vi "GTcode_v6.vi"() -> ()   [LabVIEW 2016]
uses:
  <vilib>/Utility/error.llb/DialogType.ctl
  <vilib>/Analysis/5stat.llb/RMS (DBL).vi
  <vilib>/Utility/config.llb/Write Key (String).vi
  <vilib>/Utility/config.llb/Write Key (U32).vi
  <vilib>/Utility/config.llb/Write Key (Double).vi
  <vilib>/Utility/config.llb/Write Key (I32).vi
  <vilib>/Utility/config.llb/Read Key (U32).vi
  <vilib>/Utility/config.llb/Read Key (I32).vi
  <vilib>/Waveform/WDTFileIO.llb/ Write Waveform to File.vi
  <vilib>/Waveform/WDTOps.llb/WDT Append Waveforms DBL.vi
  DCScode_simulISS_MAP/flex05-4chPascal.dll
  <vilib>/Utility/config.llb/NI_LVConfig.lvlib
  DCScode_simulISS_MAP/flex05oem8chauto100nsPASCAL_win7.dll
  <vilib>/Analysis/NI_AALBase.lvlib
  <vilib>/Analysis/NI_AALPro.lvlib
  <resource>/objmgr/daqmx.rc
panel:
  in  "Tab Control":T1(tab)=enum."Real Time Fitting Parameters"
  out "mean":dbl format="%0.1e"
  out "COV":dbl format="%0.1f"
  in  "Fixed Time":bool
  in  "Detector Used":T2(ring)=enum."Det 2"
  in  "Real Time Fitting?":bool=TRUE
  out "g2":cluster{"Delay Time":sgl[], sgl[]}[](graph) caption="Normalized Correlation Function"
  out "Tau":cluster{"tmp":dbl, dbl}(graph) caption="Relative Changes of Flow"
  in  "QUIT":bool
  in  "Clear plots":bool
  in  "Baseline":bool
  in  "MARK\nMark":bool
  in  "Stop":bool
  in  "Sequence Scan":bool
  out "Mark #":u32
  out "Trial #":u32
  out "Frame #":u32
  out "Det 8":sgl format="%.3f"
  out "Det 7":sgl format="%.3f"
  out "Det 6":sgl format="%.3f"
  out "Det 5":sgl format="%.3f"
  out "Det 4":sgl format="%.3f"
  out "Det 3":sgl format="%.3f"
  out "Det 2":sgl format="%.3f"
  out "Det 1":sgl format="%.3f"
  out "Computer Time":string="2010-1-12 23:16:10"
  in  "D1":bool
  in  "D2":bool
  in  "D3":bool
  in  "D4":bool
  in  "D5":bool
  in  "D6":bool
  in  "D7":bool
  in  "D8":bool
  out "Tau 2":T3(graph)={1.6593152555505744e-08, 3.9427894777554196e-08, 4.065716407938411e-08, 1.5135790977358522e-08, 2.4870420100428357e-08, 7.094765128107397e-08, 0.0, 4.1348620928852906e-07, 1.5886917674344795e-08, 4.0280526032721455e-08, -1.0, -1.0} caption="Blood Flow Index (cm2/s)"
  in  "Fixed # of Frames":u32=5
  out "Status":string="Quit"
  in  "Optical Switch OPEN":bool
  in  "Delay between frames(ms)":u32=500
  out "Time Left (ms)":sgl format="%.3f"
  in  "Integration Time (ms)":sgl=1000.0 min=1 max=13000 step=1
  in  "File\nName:":string="test0"
  in  "Data Save Directory:":path=path "C:/data"
  in  "ISS Lasers ON":bool
  in  "Test":bool=TRUE
  out "Moving Avg RMS":dbl(slide) scale=0.0..0.07
  out "Moving Avg RMS Graph":dbl(graph)
  out "raw data":dynamicdata(graph)
  out "Trial Data 2":waveform(dbl)(graph)
  out "Reset Data Acquisition\nAnd UI Updating":bool=TRUE
  out "Trial In Progress":bool
  in  "Lines":tag="Dev1/port1/line0:1, Dev1/port1/line3:7"
  in  "Delaytime(ms)":u32=200
  in  "Initialize Correlator":bool
  in  "Detector Select":enum32{"4 Detectors", "8 Detectors"}(radio)=enum."8 Detectors"
  in  "Update Time (ms)\nDO NOT CHANGE!":u32=105 min=1 max=999 step=1
  in  "Laser Input Name":refnum<visa-resource-name>="COM7"
  out "Flow in each detector":dbl[](array[numeric])=[-1.0, -1.0, -1.0, -1.0, -1.0, -1.0, -1.0, -1.0, -1.0, -1.0, -1.0, -1.0]
  in  "Visible Averages":bool[](array[boolean])=[FALSE, FALSE, FALSE, FALSE]
  in  "Avg":bool[][](array[boolean])=[[FALSE, FALSE, FALSE, FALSE, FALSE, FALSE, FALSE, FALSE], [FALSE, FALSE, FALSE, FALSE, FALSE, FALSE, FALSE, FALSE], [FALSE, FALSE, FALSE, FALSE, FALSE, FALSE, FALSE, FALSE], [FALSE, FALSE, FALSE, FALSE, FALSE, FALSE, FALSE, FALSE]]
  in  "rho":dbl[](array[numeric])=[2.5, 2.5, 2.5, 2.5, 2.5, 2.5, 2.5, 2.5, -1.0, -1.0, -1.0, -1.0]
  in  "Other Settings":u32[](array[numeric])=[1, 120, 0, 1] caption="Flow in each detector"
  in  "Initial Guess":dbl[](array[numeric])=[1e-08, 0.5, 0.05, 10.0] caption="Flow in each detector"
  out "Filtered data":waveform(dbl)
  out "Aggregate Data":waveform(dbl)[](array[waveform])
  in  "VR Data Input File":path
  in  "Trial Number":dbl
  in  "Target Percentage":dbl
  in  "VR Percent Path":path
  out "Trial Data":waveform(dbl)
  out "Rectified Moving Average Sample":waveform(dbl)[](graph)
  out "Bufffer Index":dbl
  out "Frames in Buffer":dbl
  out "Samples per frame":dbl
  in  "Lower Cut-Off":dbl=20.0
  in  "Upper Cut-Off (Not In Use)":dbl=300.0 caption="Upper Cut-Off"
  in  "File Name:":string="test0"
  in  "Sample rate (Hz)":dbl=2000.0
  in  "Frames Per Second":dbl=30.0
  in  "Moving Average Length (s)":dbl=0.5
  in  "EMG Input Device\nProduct Type":string
  out "4CH?":bool
  out "Detector#":u32=1
  out "Source#":u32=1
  # "Jake Test Version"
  # "kHz"
  # "kHz"
  # "Don't Change these Parameters unless you know clearly what you are doing"
  # "ISS Triggers Setup"
  # "Channel Parameters"
  # "Step1"
  # "Line"
  # "0"
  # "1"
  # "3"
  # "4"
  # "5"
  # "6"
  # "7"
  # "*The number of lines in the list must\nmatch the number of elements in\nthe array."
  # "Step2"
  # "Line"
  # "0"
  # "1"
  # "3"
  # "4"
  # "5"
  # "6"
  # "7"
  # "Step3"
  # "Line"
  # "0"
  # "1"
  # "3"
  # "4"
  # "5"
  # "6"
  # "7"
  # "Line    Signal\n\n0           ISS Trigger (0: OFF, 1: ON)\n1           Flow Laser 1 ON/OFF (0:OFF, 1:ON)\n2           ISS Data Acquisition (0: DONE, 1: NO)\n3           ISS Laser ON/OFF (0: ON, 1: OFF)\n4           Trigger for Marks  (0: OFF, 1: ON)\n5           Flow Laser 2 ON/OFF (0:OFF, 1:ON)\n6           Reserved\n7           Reserved"
  # "Wait ISS Data Acuisition DONE Signal"
  # "Step4"
  # "Step5"
  # "Line"
  # "0"
  # "1"
  # "3"
  # "4"
  # "5"
  # "6"
  # "7"
  # "Flow Lasers Setup"
  # "FROM FRONT PANEL"
  # "Line"
  # "0"
  # "1"
  # "3"
  # "4"
  # "5"
  # "6"
  # "7"
  # "Line"
  # "0"
  # "1"
  # "3"
  # "4"
  # "5"
  # "6"
  # "7"
  # "Det 1"
  # "Det 2"
  # "Det 3"
  # "Det 4"
  # "Det 5"
  # "Det 6"
  # "Det 7"
  # "Det 8"
  # "Avg 1"
  # "Avg 2"
  # "Avg 3"
  # "Avg 4"
  # "Db"
  # "Beta"
  # "Mua"
  # "MuS'"
  # "1"
  # "2"
  # "3"
  # "4"
  # "5"
  # "6"
  # "7"
  # "8"
  # "Avg 1"
  # "Starting Pt"
  # "End Pt"
  # "Approximate"
  # "Variables"
  # "Avg 2"
  # "Avg 3"
  # "Avg 4"
  # "Source Detector  Separations"
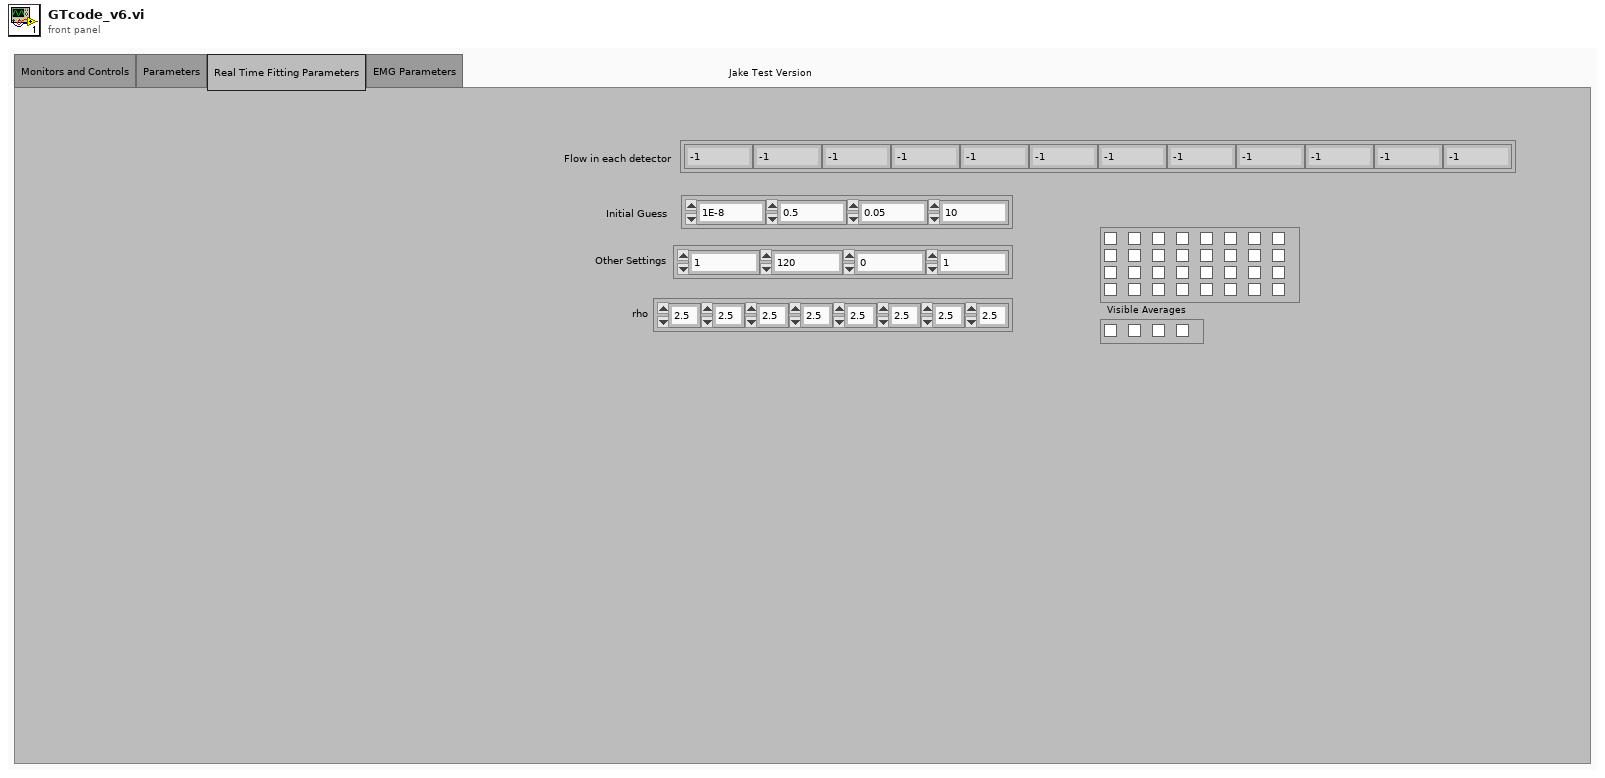
[diagram p1: front panel]
types:
  T1 = enum32{"Monitors and Controls", "Parameters", "Real Time Fitting Parameters", "EMG Parameters"}
  T2 = enum16{"Det 1", "Det 2", "Det 3", "Det 4", "Det 5", "Det 6", "Det 7", "Det 8"}
  T3 = cluster{dbl, dbl, dbl, dbl, dbl, dbl, dbl, dbl, dbl, dbl, dbl, dbl}
  T4 = typedef "DialogType.ctl" = u16
  T5 = enum8{"Enabled", "Disabled", "Disabled and Grayed Out"}
  T6 = cluster{dbl, dbl, dbl, dbl, dbl, dbl, dbl, dbl, dbl, dbl, dbl, dbl}[]
  T7 = typedef "NI_LVConfig.lvlib/Config Data RefNum.ctl" = refnum<k1>
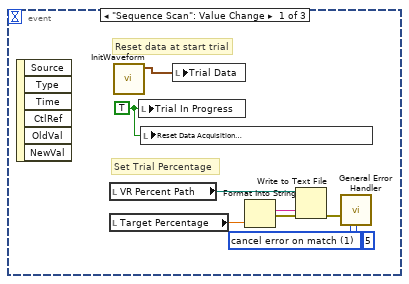
[diagram p2: hidden frame]
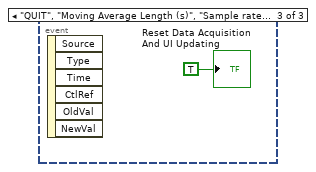
[diagram p5: hidden frame]
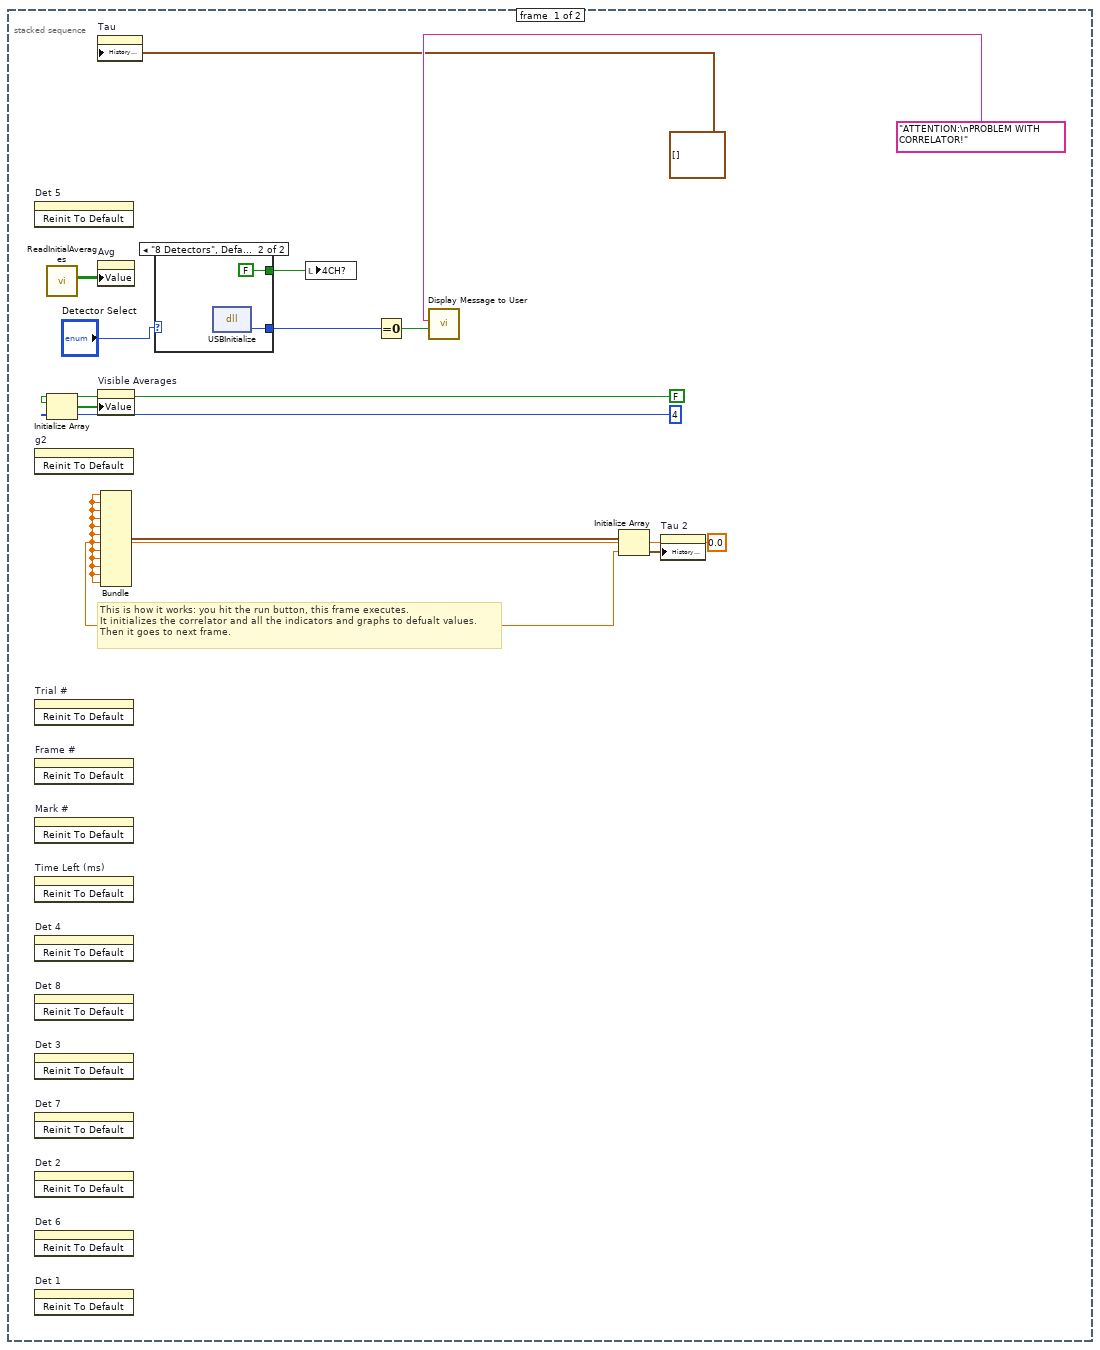
[diagram p7: hidden frame]
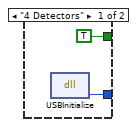
[diagram p8: hidden frame]
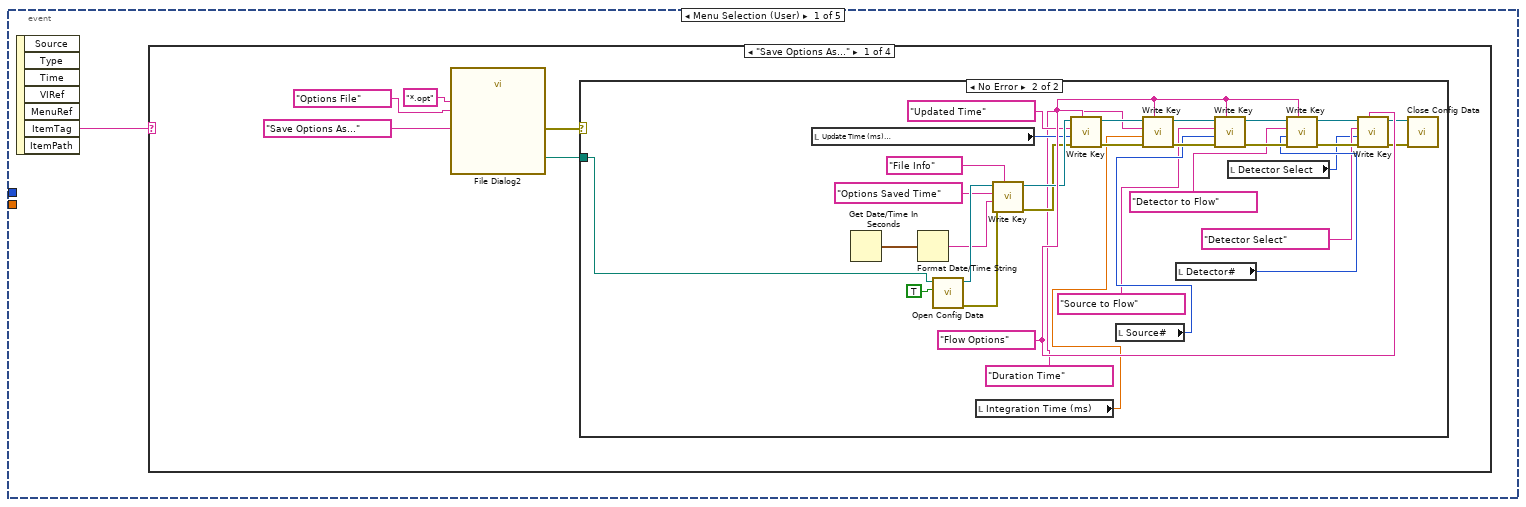
[diagram p10: hidden frame]
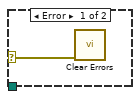
[diagram p11: hidden frame]
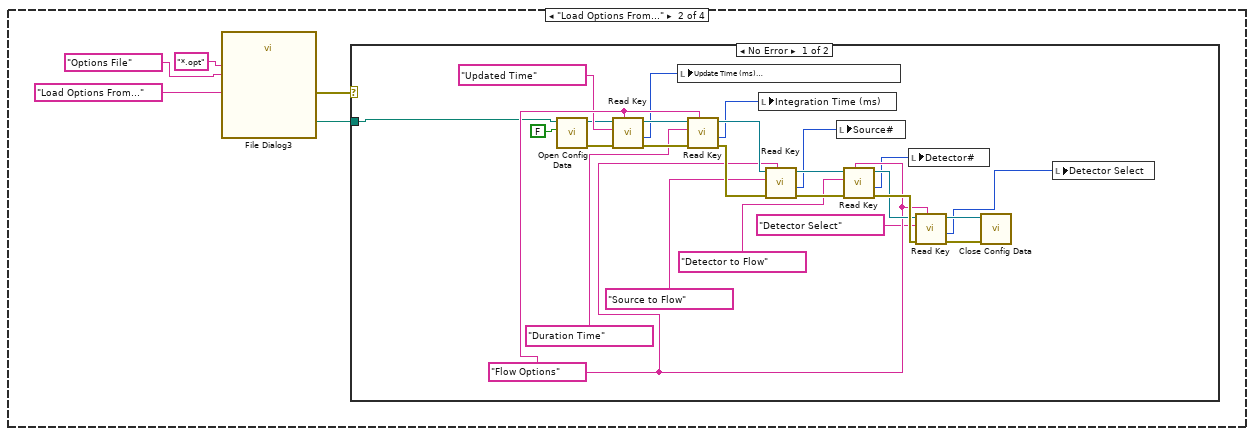
[diagram p12: hidden frame]
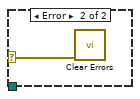
[diagram p13: hidden frame]
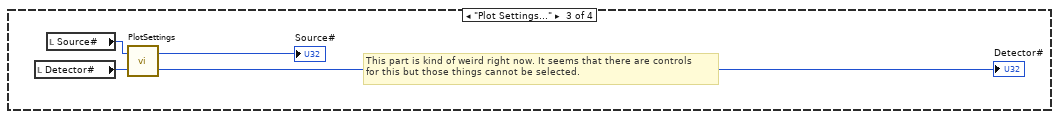
[diagram p14: hidden frame]
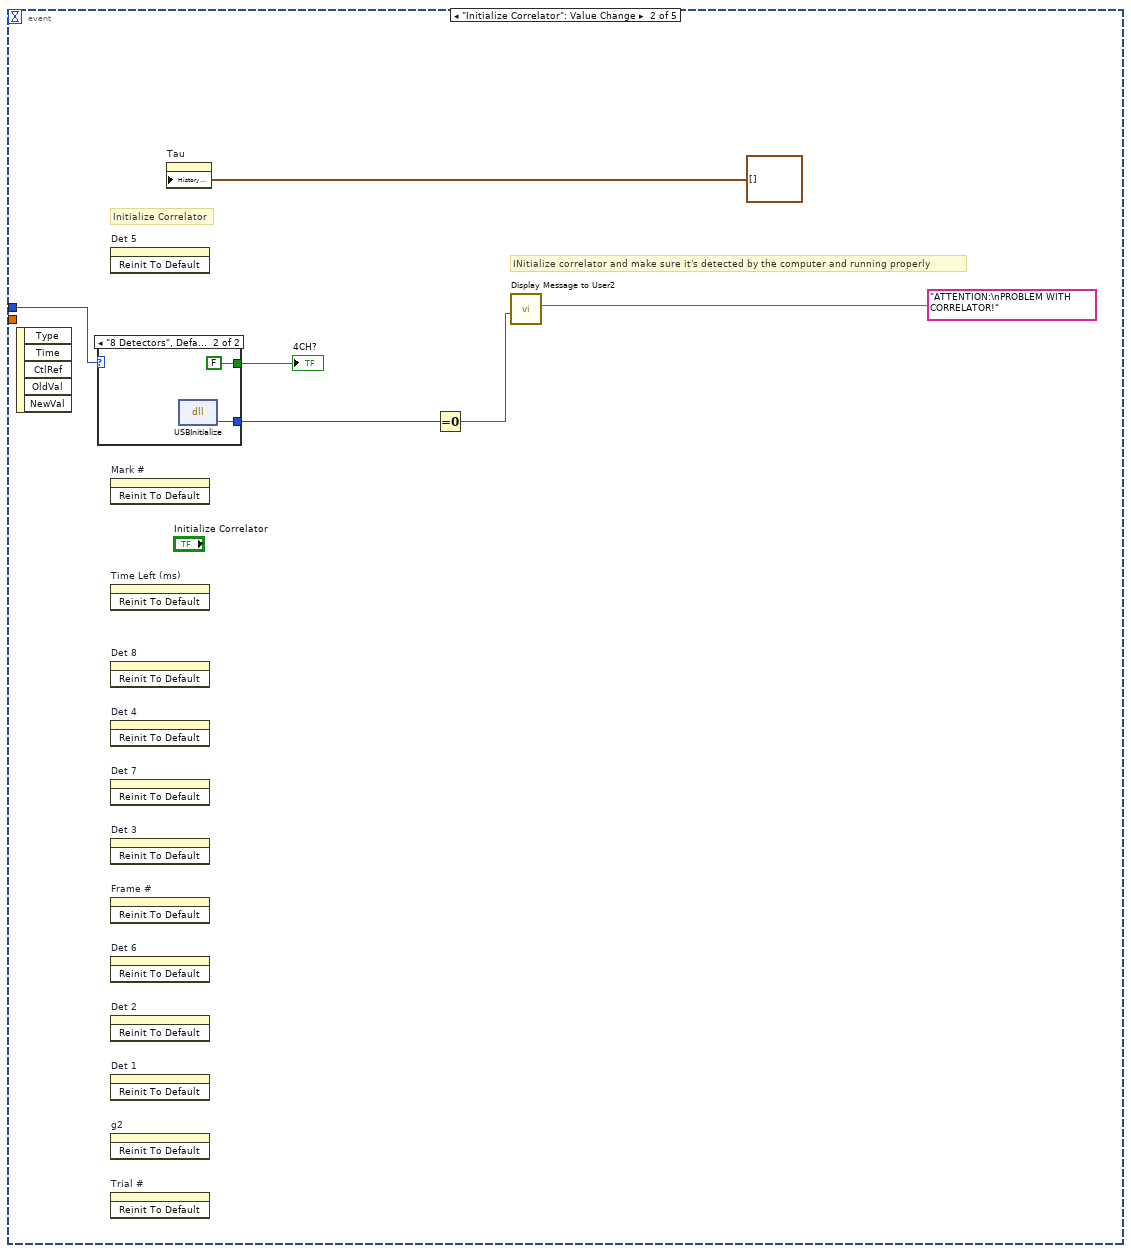
[diagram p16: hidden frame]
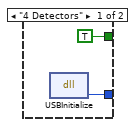
[diagram p17: hidden frame]
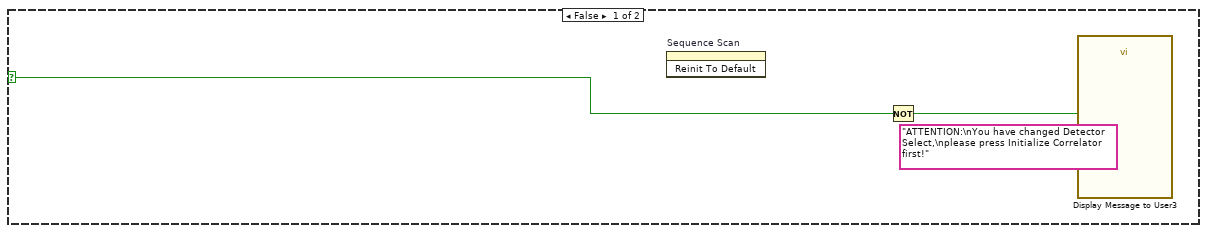
[diagram p18: hidden frame]
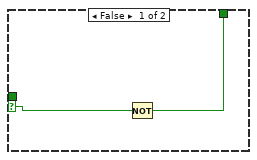
[diagram p19: hidden frame]
diagram:
  # "Where VR knows\n to look for data"
  n1 = property class="DAQmx System"() -> ("DevNames"=w2:tag[])  [unwired: 2 in, 2 out]
  n2 = for {
    tunnel: w2 -> [w6] mode=indexing
    tunnel: [w6] -> w1
    stop <- w7 stop-if-true
    n3 = property class="DAQmx Device" props=["Active Device", "ProductType", "ProductNum"]("Active Device"=w6) -> ("ProductType"=w9:string)  [unwired: 2 in, 3 out]
    n4 = Equal?(x=w9, y="EMG Input Device\nProduct Type") -> (x = y?=w7:bool)
  }
  n5 = while {
    tunnel: w1 -> [w10]
    stop <- w11 stop-if-true
    # "Initialize Stuff"
    # "Listen for settings changes and restart runtime loop\nAlso make updates for trial changes"
    n6 = while {
      tunnel: w10 -> [w62]
      stop <- w65 stop-if-true
      n7 = local read "Sample rate (Hz)"() -> (w79:dbl)
      n8 = local read "Samples per frame"() -> (w78:dbl)
      n9 = local read "Reset Data Acquisition\nAnd UI Updating"() -> (w64:bool)
      n10 = local read "raw data"() -> (w76:dynamicdata)
      n11 = local read "Aggregate Data"() -> (w72:waveform(dbl)[])
      n12 = local read "Filtered data"() -> (w71:waveform(dbl))
      n13 = local read "Bufffer Index"() -> (w70:dbl)
      n14 = local read "Frames in Buffer"() -> (w67:dbl)
      n15 = local read "Trial In Progress"() -> (w63:bool)
      n16 = local read "Reset Data Acquisition\nAnd UI Updating"() -> (w65:bool)
      n17 = case shown="True" w63 {
        frame False {
        }
        frame True {
          # "Start aggregating data for trial"
          n18 = local read "Filtered data"() -> (w81:waveform(dbl))
          n19 = local read "Trial Data"() -> (w82:waveform(dbl))
          n20 = call-poly <vilib>:"Append Waveforms.vi"("waveform B"=w81, "waveform A"=w82) -> ("waveform out"=w80:waveform(dbl))  [unwired: 8 in, 1 out]
          n21 = local write "Trial Data"(w80) -> ()
        }
      }
      n22 = call "Filter"("Lower Cut-Off"="Lower Cut-Off", "Signal"=w76) -> ("Filtered Signal"=w74:dynamicdata)  [unwired: 8 in, 1 out]
      n23 = Increment(x=w70) -> (x+1=w66:dbl)
      n24 = Replace Array Subset(array=w72, new element=w71, index=w70) -> (w69:waveform(dbl)[])
      n25 = call "DAQ Assistant8"("rate"=w79, "number of samples"=w78, "stop (T)"=w64, "device name"=w62) -> ("data"=→"raw data":dynamicdata)  [unwired: 13 in, 2 out]
      n26 = Quotient & Remainder(x=w66, y=w67) -> (x-y*floor(x/y)=w68:dbl)  [unwired: 1 out]
      n27 = local write "Aggregate Data"(w69) -> ()
      n28 = call "Convert from Dynamic Data"("Dynamic Data Type"=w74) -> ("Waveform"=→"Filtered data":waveform(dbl))  [unwired: 3 in]
      n29 = local write "Bufffer Index"(w68) -> ()
    }
    n30 = local read "Moving Average Length (s)"() -> (w17:dbl)
    n31 = local read "Frames Per Second"() -> (w16:dbl)
    n32 = local read "QUIT"() -> (w11:bool)
    n33 = local read "Sample rate (Hz)"() -> (w20:dbl)
    n34 = local read "Frames Per Second"() -> (w19:dbl)
    n35 = local write "Reset Data Acquisition\nAnd UI Updating"(FALSE) -> ()
    n36 = Divide(x=w20, y=w19) -> (x/y=→"Samples per frame":dbl)
    n37 = Multiply(x=w17, y=w16) -> (x*y=w12:dbl)
    "Frames in Buffer" <- w12
    n38 = call "CreateWaveformArray.vi"("bufferSize"=w12) -> ("initialized array"=→"Aggregate Data":waveform(dbl)[])  [unwired: 5 in, 1 out]
    n39 = event shown="[1] \"Stop\": Value Change" {
      selector: _ -> [_ _ _]
      dyn-events: _ -> [_ _ _]
      timeout: _ -> [_ _ _]
      event "Sequence Scan": Value Change {
        w27 = 1 items=["no exception", "cancel error on match", "set error on match"] ("[exception action] (none:0)")
        w28 = TRUE ("Trial In Progress")
        # "Set Trial Percentage"
        # "Reset data at start trial"
        n40 = event-data() -> ()  [unwired: 1 in, 6 out]
        n41 = local read "VR Percent Path"() -> (w22:path)
        n42 = local read "Target Percentage"() -> (w21:dbl)
        n43 = call "InitWaveform.vi"() -> ("output waveform"=w29:waveform(dbl))  [unwired: 11 in]
        n44 = local write "Trial In Progress"(w28) -> ()
        n45 = local write "Reset Data Acquisition\nAnd UI Updating"(w28) -> ()
        n46 = local write "Trial Data"(w29) -> ()
        n47 = Format Into String(w21) -> (resulting string=w23:string, error out=w24:errorcluster)  [unwired: 3 in]
        n48 = Write to Text File(file (use dialog)=w22, text=w23, error in=w24) -> (error out=w25:errorcluster)  [unwired: 1 in, 2 out]
        n49 = call <vilib>:"General Error Handler.vi"("error in (no error)"=w25, "[exception action] (none:0)"=w27, "[exception code]"=5) -> ()  [unwired: 8 in, 5 out]
      }
      event "Stop": Value Change {
        # "Only Execute if Trial Already in progress"
        n50 = event-data() -> ()  [unwired: 1 in, 6 out]
        n51 = local read "Trial In Progress"() -> (w30:bool)
        n52 = case shown="True" w30 {
          frame False {
          }
          frame True {
            w31 = T4 2 items=["no dialog", "OK message", "continue or stop message", "OK message + warnings", "continue/stop + warnings"] ("type of dialog (OK msg:1)")
            w33 = 1 items=["no exception", "cancel error on match", "set error on match"] ("[exception action] (none:0)")
            # "End Trial and save data, create directory if needed"
            n53 = local read "Data Save Directory:"() -> (w38:path)
            n54 = local read "Trial Data"() -> (w45:waveform(dbl))
            n55 = local read "File Name:"() -> (w37:string)
            n56 = local write "Trial In Progress"(FALSE ("Trial In Progress")) -> ()
            n57 = local write "Reset Data Acquisition\nAnd UI Updating"(TRUE ("Reset Data Acquisition\nAnd UI Updating")) -> ()
            n58 = Concatenate Strings(w37, "_EMG.dat" ("string")) -> (w35:string)
            n59 = call <vilib>:"Check if File or Folder Exists.vi"("path"=w38) -> ("file or folder exists?"=w42:bool, "dup path"=w40:path)  [unwired: 8 in, 1 out]
            n60 = case shown="False" w42 {
              tunnel: [w47 w49] -> w41
              tunnel: w40 -> [w48 w49]
              frame False {
                n61 = Create Folder(path (use dialog)=w48) -> (created path=w47:path)  [unwired: 2 in, 2 out]
              }
              frame True {
              }
            }
            n62 = Build Path(base path=w41, name or relative path=w35) -> (appended path=w39:path)
            n63 = call-poly <vilib>:"Write Waveforms to File.vi"("append to file? (new file:F)"=FALSE, "waveform"=w45, "file path (dialog if empty)"=w39) -> ("error out"=w32:errorcluster)  [unwired: 7 in, 1 out]
            n64 = call <vilib>:"General Error Handler.vi"("type of dialog (OK msg:1)"=w31, "error in (no error)"=w32, "[exception action] (none:0)"=w33, "[exception code]"=1430) -> ()  [unwired: 7 in, 5 out]
          }
        }
      }
      event "QUIT", "Moving Average Length (s)", "Sample rate (Hz)", "Frames Per Second": Value Change {
        n65 = event-data() -> ()  [unwired: 1 in, 6 out]
        "Reset Data Acquisition\nAnd UI Updating" <- TRUE
      }
    }
    n66 = while {
      stop <- w61 stop-if-true
      # "Grab Relevant Sample from Moving Average, Update UI, Save Data if necessary"
      # "Wait proper duration"
      # "Save RMS Value\nFor this Frame To VR"
      # "Display RMS Data\nTo Thermometer\nAnd Moving Avg RMS\nGraph"
      # "Grab Current Moving\nAverage and Rectify"
      # "Get Moving Average Sample"
      # "Rectify"
      n67 = local read "Rectified Moving Average Sample"() -> (w58:waveform(dbl)[])
      n68 = local read "Bufffer Index"() -> (w53:dbl)
      n69 = local read "Frames in Buffer"() -> (w52:dbl)
      n70 = local read "Aggregate Data"() -> (w51:waveform(dbl)[])
      n71 = local read "Frames Per Second"() -> (w57:dbl)
      n72 = local read "Reset Data Acquisition\nAnd UI Updating"() -> (w61:bool)
      n73 = call "FramesPerSecondTOMilliseconds.vi"("Thermometer\nFps"=w57) -> ("x*y"=w56:dbl)  [unwired: 10 in]
      n74 = call "GetSubarrayOfCircularBuffer.vi"("initialized array"=w51, "buffer size"=w52, "subset size"=w52, "start index"=w53) -> ("initialized array 2"=w54:waveform(dbl)[])  [unwired: 7 in]
      n75 = Wait (ms)(milliseconds to wait=w56) -> ()  [unwired: 1 out]
      n76 = local read "Trial Data"() -> (→"Trial Data 2":waveform(dbl))
      n77 = Absolute Value(x=w54) -> (abs(x)=→"Rectified Moving Average Sample":waveform(dbl)[])
      n78 = call-poly <vilib>:"RMS.vi"("X"=w58) -> ("rms value"=→"Moving Avg RMS" →"Moving Avg RMS Graph":dbl)  [unwired: 1 out]
    }
    "Bufffer Index" <- 0.0 ("Bufffer Index")
  }
  n79 = local read "Laser Input Name"() -> (w4:refnum<visa-resource-name>)
  n80 = call "iBs.vi"("Laser On/Off"=FALSE, "VISA resource name"=w4) -> ()
  n81 = stacked-sequence {
    frame #0 {
      w85 = 0.0
      # "This is how it works: you hit the run button, this frame executes.\nIt initializes the correlator and all the indicators and graphs to defualt values.\nThen it goes to next frame."
      n82 = invoke on="Det 5" class="DigNum (strict)" method="Reinit To Default"() -> ()  [unwired: 3 in, 3 out]
      n83 = invoke on="g2" class="XYGraph (strict)" method="Reinit To Default"() -> ()  [unwired: 3 in, 3 out]
      n84 = invoke on="Trial #" class="DigNum (strict)" method="Reinit To Default"() -> ()  [unwired: 3 in, 3 out]
      n85 = invoke on="Frame #" class="DigNum (strict)" method="Reinit To Default"() -> ()  [unwired: 3 in, 3 out]
      n86 = invoke on="Mark #" class="DigNum (strict)" method="Reinit To Default"() -> ()  [unwired: 3 in, 3 out]
      n87 = invoke on="Time Left (ms)" class="DigNum (strict)" method="Reinit To Default"() -> ()  [unwired: 3 in, 3 out]
      n88 = invoke on="Det 4" class="DigNum (strict)" method="Reinit To Default"() -> ()  [unwired: 3 in, 3 out]
      n89 = invoke on="Det 8" class="DigNum (strict)" method="Reinit To Default"() -> ()  [unwired: 3 in, 3 out]
      n90 = invoke on="Det 3" class="DigNum (strict)" method="Reinit To Default"() -> ()  [unwired: 3 in, 3 out]
      n91 = invoke on="Det 7" class="DigNum (strict)" method="Reinit To Default"() -> ()  [unwired: 3 in, 3 out]
      n92 = invoke on="Det 2" class="DigNum (strict)" method="Reinit To Default"() -> ()  [unwired: 3 in, 3 out]
      n93 = invoke on="Det 6" class="DigNum (strict)" method="Reinit To Default"() -> ()  [unwired: 3 in, 3 out]
      n94 = invoke on="Det 1" class="DigNum (strict)" method="Reinit To Default"() -> ()  [unwired: 3 in, 3 out]
      n95 = call "ReadInitialAverages.vi"() -> ("avgOut"=w84:bool[][])  [unwired: 11 in]
      n96 = Initialize Array(FALSE, 4) -> (w83:bool[])
      n97 = property on="Tau" class="WFChart (strict)"("History Data"=cluster{"tmp":dbl, dbl}[] []) -> ()  [unwired: 2 in, 2 out]
      n98 = property on="Avg" class="Arr (strict)"("Value"=w84) -> ()  [unwired: 2 in, 2 out]
      n99 = property on="Visible Averages" class="Arr (strict)"("Value"=w83) -> ()  [unwired: 2 in, 2 out]
      n100 = Bundle(w85, w85, w85, w85, w85, w85, w85, w85, w85, w85, w85, w85) -> (w87:T3)  [unwired: 1 in]
      n101 = case shown="\"8 Detectors\", Default" "Detector Select" {
        tunnel: [w97 w99] -> w95
        tunnel: [TRUE FALSE] -> w93
        frame "4 Detectors" {
          n102 = dll-call lib="C:/Users/BUCKLEY-ADMIN/Desktop/DCScode_simulISS_MAP/flex05-4chPascal.dll" fn="USBInitialize" label="InitCH4"() -> ("return type"=w97:u8)  [unwired: 3 in, 2 out]
        }
        frame "8 Detectors", Default {
          n103 = dll-call lib="C:/Users/BUCKLEY-ADMIN/Desktop/DCScode_simulISS_MAP/flex05oem8chauto100nsPASCAL_win7.dll" fn="USBInitialize" label="InitCH8"() -> ("return type"=w99:u8)  [unwired: 3 in, 2 out]
        }
      }
      n104 = local write "4CH?"(w93) -> ()
      n105 = Equal To 0?(x=w95) -> (x = 0?=w94:bool)
      n106 = call "Display Message to User"("Enable"=w94, "Message"="ATTENTION:\nPROBLEM WITH CORRELATOR!") -> ()  [unwired: 8 in, 2 out]
      n107 = Initialize Array(w87, w85) -> (w86:T6)
      n108 = property on="Tau 2" class="WFChart (strict)"("History Data"=w86) -> ()  [unwired: 2 in, 2 out]
    }
    frame #1 {
      n109 = while {
        stop <- w103 stop-if-true
        # "Looks at whether using 4 or 8 ch correlator\nGenerates time points for g2 function based on correlator"
        n110 = local read "Detector Select"() -> (w101:enum32{"4 Detectors", "8 Detectors"})
        n111 = case shown="\"8 Detectors\"" w101 {
          tunnel: [_ w104] -> w100
          frame "4 Detectors", Default {
          }
          frame "8 Detectors" {
            n112 = formula code="int i,j;\nfloat DelayTime[256];\nfloat first_delay;\n\nfirst_delay = 2E-7;\n\nfor(i=0;i<16;i++)\nDelayTime[i] = (i+1)*first_delay;\nfor(j=1;j<31;j++)\n    for(i=0;i<8;i++)\n         DelayTime[i+(j-1)*8+16] = DelayTime[(j-1)*8+16+i-1]+first_delay*pow(2,j);"() -> ("DelayTime"=w104:dbl[])
          }
        }
        n113 = event shown="[2] \"Sequence Scan\": Value Change" {
          selector: _ -> [_ _ _ _ _]
          dyn-events: _ -> [_ _ _ _ _]
          timeout: 500 -> [_ _ _ _ _]
          tunnel: w100 -> [_ _ w194 _ _]
          tunnel: [_ _ _ "QUIT" _] -> w103
          tunnel: w101 -> [_ w181 w190 w678 _]
          event Menu Selection (User) {
            n114 = event-data() -> ("ItemTag"=w105:string)  [unwired: 1 in, 6 out]
            n115 = case shown="\"Save Options As...\"" w105 {
              frame "Save Options As..." {
                n116 = call "File Dialog2"("prompt"="Save Options As...", "pattern (all files)"="*.opt", "pattern label"="Options File") -> ("selected path"=w107:path, "error out"=w106:errorcluster)  [unwired: 9 in, 2 out]
                n117 = case shown="No Error" w106 {
                  selector: w106 -> [w111 _]
                  tunnel: w107 -> [_ w142]
                  frame Error {
                    n118 = call <vilib>:"Clear Errors.vi"("error in (no error)"=w111) -> ()  [unwired: 5 in, 2 out]
                  }
                  frame No Error {
                    w129 = "Flow Options"
                    n119 = local read "Update Time (ms)\nDO NOT CHANGE!"() -> (w122:u32)
                    n120 = Get Date/Time In Seconds() -> (seconds since 1Jan1904=w128:timestamp)
                    n121 = Format Date/Time String(seconds (now)=w128) -> (date/time string=w124:string)  [unwired: 2 in]
                    n122 = call <vilib>:"Open Config Data.vi"("create file if necessary (T)"=TRUE, "configuration file path"=w142) -> ("error out"=w140:errorcluster, "refnum"=w139:T7)  [unwired: 7 in, 1 out]
                    n123 = local read "Integration Time (ms)"() -> (w120:sgl)
                    n124 = call-poly <vilib>:"Write Key.vi"("section"="File Info", "error in (no error)"=w140, "value"=w124, "key"="Options Saved Time", "refnum"=w139) -> ("error out"=w126:errorcluster, "refnum out"=w127:T7)  [unwired: 4 in, 1 out]
                    n125 = call-poly <vilib>:"Write Key.vi"("section"=w129, "error in (no error)"=w126, "value"=w122, "key"="Updated Time", "refnum"=w127) -> ("error out"=w138:errorcluster, "refnum out"=w137:T7)  [unwired: 4 in, 1 out]
                    n126 = local read "Source#"() -> (w119:u32)
                    n127 = call-poly <vilib>:"Write Key.vi"("section"=w129, "error in (no error)"=w138, "value"=w120, "key"="Duration Time", "refnum"=w137) -> ("error out"=w133:errorcluster, "refnum out"=w134:T7)  [unwired: 4 in, 1 out]
                    n128 = local read "Detector#"() -> (w116:u32)
                    n129 = call-poly <vilib>:"Write Key.vi"("section"=w129, "error in (no error)"=w133, "value"=w119, "key"="Source to Flow", "refnum"=w134) -> ("error out"=w135:errorcluster, "refnum out"=w136:T7)  [unwired: 4 in, 1 out]
                    n130 = local read "Detector Select"() -> (w114:enum32{"4 Detectors", "8 Detectors"})
                    n131 = call-poly <vilib>:"Write Key.vi"("section"=w129, "error in (no error)"=w135, "value"=w116, "key"="Detector to Flow", "refnum"=w136) -> ("error out"=w132:errorcluster, "refnum out"=w131:T7)  [unwired: 4 in, 1 out]
                    n132 = call-poly <vilib>:"Write Key.vi"("section"=w129, "error in (no error)"=w132, "value"=w114, "key"="Detector Select", "refnum"=w131) -> ("error out"=w112:errorcluster, "refnum out"=w113:T7)  [unwired: 4 in, 1 out]
                    n133 = call <vilib>:"Close Config Data.vi"("error in (no error)"=w112, "refnum"=w113) -> ()  [unwired: 8 in, 2 out]
                  }
                }
              }
              frame "Load Options From..." {
                n134 = call "File Dialog3"("prompt"="Load Options From...", "pattern (all files)"="*.opt", "pattern label"="Options File") -> ("selected path"=w144:path, "error out"=w143:errorcluster)  [unwired: 9 in, 2 out]
                n135 = case shown="No Error" w143 {
                  selector: w143 -> [_ w173]
                  tunnel: w144 -> [w148 _]
                  frame No Error {
                    w163 = "Flow Options"
                    n136 = call <vilib>:"Open Config Data.vi"("create file if necessary (T)"=FALSE, "configuration file path"=w148) -> ("error out"=w155:errorcluster, "refnum"=w154:T7)  [unwired: 7 in, 1 out]
                    n137 = call-poly <vilib>:"Read Key.vi"("section"=w163, "error in (no error)"=w155, "key"="Updated Time", "refnum"=w154) -> ("error out"=w171:errorcluster, "value"=w153:u32, "refnum out"=w170:T7)  [unwired: 4 in, 1 out]
                    n138 = local write "Update Time (ms)\nDO NOT CHANGE!"(w153) -> ()
                    n139 = call-poly <vilib>:"Read Key.vi"("section"=w163, "error in (no error)"=w171, "key"="Duration Time", "refnum"=w170) -> ("error out"=w166:errorcluster, "value"=w152:i32, "refnum out"=w167:T7)  [unwired: 4 in, 1 out]
                    n140 = local write "Integration Time (ms)"(w152) -> ()
                    n141 = call-poly <vilib>:"Read Key.vi"("section"=w163, "error in (no error)"=w166, "key"="Source to Flow", "refnum"=w167) -> ("error out"=w168:errorcluster, "value"=w149:u32, "refnum out"=w169:T7)  [unwired: 4 in, 1 out]
                    n142 = local write "Source#"(w149) -> ()
                    n143 = call-poly <vilib>:"Read Key.vi"("section"=w163, "error in (no error)"=w168, "key"="Detector to Flow", "refnum"=w169) -> ("error out"=w165:errorcluster, "value"=w150:u32, "refnum out"=w164:T7)  [unwired: 4 in, 1 out]
                    n144 = local write "Detector#"(w150) -> ()
                    n145 = call-poly <vilib>:"Read Key.vi"("section"=w163, "error in (no error)"=w165, "key"="Detector Select", "refnum"=w164) -> ("error out"=w156:errorcluster, "value"=w151:u32, "refnum out"=w157:T7)  [unwired: 4 in, 1 out]
                    n146 = call <vilib>:"Close Config Data.vi"("error in (no error)"=w156, "refnum"=w157) -> ()  [unwired: 8 in, 2 out]
                    n147 = local write "Detector Select"(w151) -> ()
                  }
                  frame Error {
                    n148 = call <vilib>:"Clear Errors.vi"("error in (no error)"=w173) -> ()  [unwired: 5 in, 2 out]
                  }
                }
              }
              frame "Plot Settings..." {
                # "This part is kind of weird right now. It seems that there are controls\nfor this but those things cannot be selected."
                n149 = local read "Detector#"() -> (w175:u32)
                n150 = local read "Source#"() -> (w176:u32)
                n151 = call "PlotSettings.vi"("Detectorin"=w175, "Sourcein"=w176) -> ("Detector#"=→"Detector#":u32, "Source#"=→"Source#":u32)
              }
              frame Default {
              }
            }
          }
          event "Initialize Correlator": Value Change {
            # "INitialize correlator and make sure it's detected by the computer and running properly"
            # "Initialize Correlator"
            n152 = event-data() -> ()  [unwired: 1 in, 5 out]
            n153 = case shown="\"8 Detectors\", Default" w181 {
              tunnel: [w185 w187] -> w183
              tunnel: [TRUE FALSE] -> w180
              frame "4 Detectors" {
                n154 = dll-call lib="C:/Users/BUCKLEY-ADMIN/Desktop/DCScode_simulISS_MAP/flex05-4chPascal.dll" fn="USBInitialize" label="InitCH4"() -> ("return type"=w185:u8)  [unwired: 3 in, 2 out]
              }
              frame "8 Detectors", Default {
                n155 = dll-call lib="C:/Users/BUCKLEY-ADMIN/Desktop/DCScode_simulISS_MAP/flex05oem8chauto100nsPASCAL_win7.dll" fn="USBInitialize" label="InitCH8"() -> ("return type"=w187:u8)  [unwired: 3 in, 2 out]
              }
            }
            "4CH?" <- w180
            n156 = invoke on="Det 5" class="DigNum (strict)" method="Reinit To Default"() -> ()  [unwired: 3 in, 3 out]
            n157 = invoke on="Mark #" class="DigNum (strict)" method="Reinit To Default"() -> ()  [unwired: 3 in, 3 out]
            n158 = invoke on="Time Left (ms)" class="DigNum (strict)" method="Reinit To Default"() -> ()  [unwired: 3 in, 3 out]
            n159 = invoke on="Det 8" class="DigNum (strict)" method="Reinit To Default"() -> ()  [unwired: 3 in, 3 out]
            n160 = invoke on="Det 4" class="DigNum (strict)" method="Reinit To Default"() -> ()  [unwired: 3 in, 3 out]
            n161 = invoke on="Det 7" class="DigNum (strict)" method="Reinit To Default"() -> ()  [unwired: 3 in, 3 out]
            n162 = invoke on="Det 3" class="DigNum (strict)" method="Reinit To Default"() -> ()  [unwired: 3 in, 3 out]
            n163 = invoke on="Frame #" class="DigNum (strict)" method="Reinit To Default"() -> ()  [unwired: 3 in, 3 out]
            n164 = invoke on="Det 6" class="DigNum (strict)" method="Reinit To Default"() -> ()  [unwired: 3 in, 3 out]
            n165 = invoke on="Det 2" class="DigNum (strict)" method="Reinit To Default"() -> ()  [unwired: 3 in, 3 out]
            n166 = invoke on="Det 1" class="DigNum (strict)" method="Reinit To Default"() -> ()  [unwired: 3 in, 3 out]
            n167 = invoke on="g2" class="XYGraph (strict)" method="Reinit To Default"() -> ()  [unwired: 3 in, 3 out]
            n168 = invoke on="Trial #" class="DigNum (strict)" method="Reinit To Default"() -> ()  [unwired: 3 in, 3 out]
            n169 = property on="Tau" class="WFChart (strict)"("History Data"=cluster{"tmp":dbl, dbl}[] []) -> ()  [unwired: 2 in, 2 out]
            n170 = Equal To 0?(x=w183) -> (x = 0?=w182:bool)
            n171 = call "Display Message to User2"("Enable"=w182, "Message"="ATTENTION:\nPROBLEM WITH CORRELATOR!") -> ()  [unwired: 8 in, 2 out]
          }
          event "Sequence Scan": Value Change {
            # "Initialize Baseline"
            n172 = event-data() -> ()  [unwired: 1 in, 6 out]
            n173 = case shown="\"8 Detectors\", Default" w190 {
              tunnel: [w673 w674] -> w189
              frame "4 Detectors" {
                n174 = local read "4CH?"() -> (w673:bool)
              }
              frame "8 Detectors", Default {
                # "Select whether using 4 or 8ch correlator"
                n175 = local read "4CH?"() -> (w675:bool)
                n176 = Not(x=w675) -> (.not. x?=w674:bool)
              }
            }
            n177 = case shown="True" w189 {
              selector: w189 -> [w196 _]
              tunnel: w194 -> [_ w210]
              tunnel: w190 -> [_ w211]
              tunnel: sgl 1.0 -> [_ w209]
              frame False {
                n178 = invoke on="Sequence Scan" class="Bool" method="Reinit To Default"() -> ()  [unwired: 3 in, 3 out]
                n179 = Not(x=w196) -> (.not. x?=w195:bool)
                n180 = call "Display Message to User3"("Enable"=w195, "Message"="ATTENTION:\nYou have changed Detector Select,\nplease press Initialize Correlator first!") -> ()  [unwired: 8 in, 2 out]
              }
              frame True {
                # "This part pauses and alerts user that test function is on. If test function is accepted then code runs but data is not saved (no timestamp either)."
                # "This checks for if the file already exists in the directory using the timing file. \n*If YES, then we don't do anything to the lasers. We just display message and wait for the user to input a new name and press sequence again.\n*If NO, then we proceed as per normal."
                n181 = local read "File\nName:"() -> (w205:string)
                n182 = case shown="True" "Test" {
                  selector: "Test" -> [w213 _]
                  tunnel: "Test" -> [_ w215]
                  tunnel: [w212 w214] -> w198
                  frame False {
                    n183 = Not(x=w213) -> (.not. x?=w212:bool)
                  }
                  frame True {
                    n184 = call "Test ON"("Enable"=w215) -> ("No - STOP"=w216:bool, "OK"=w214:bool)  [unwired: 15 in, 2 out]
                    n185 = local write "Stop"(w216) -> ()
                  }
                }
                n186 = local read "Data Save Directory:"() -> (w204:path)
                n187 = Concatenate Strings(w205, "_TIMING", ".dat") -> (w207:string)
                n188 = Build Path(base path=w204, name or relative path=w207) -> (appended path=w203:path)
                n189 = call <vilib>:"Check if File or Folder Exists.vi"("path"=w203) -> ("file or folder exists?"=w200:bool)  [unwired: 8 in, 2 out]
                n190 = Not(x=w200) -> (.not. x?=w202:bool)
                n191 = Not And(1:w198, 2:w202) -> (0:w201:bool)
                n192 = case shown="False" w201 {
                  tunnel: w211 -> [w230 _]
                  tunnel: w210 -> [w229 _]
                  tunnel: w209 -> [w228 _]
                  frame False {
                    # "Turn relay on so that Optical switch is open and LED indicator is ON"
                    # "When the START button is pressed, the ISS lasers turn off"
                    n193 = local read "Test"() -> (w217:bool)
                    n194 = case shown="False" w217 {
                      frame False {
                        # "This bit stores the time stamp."
                        n195 = local read "File\nName:"() -> (w231:string)
                        n196 = Get Date/Time In Seconds() -> (seconds since 1Jan1904=w233:timestamp)
                        n197 = local read "Data Save Directory:"() -> (w232:path)
                        n198 = Format Date/Time String(seconds (now)=w233) -> (date/time string=w239:string)  [unwired: 2 in]
                        n199 = Concatenate Strings(w231, "_TIMING", ".dat") -> (w236:string)
                        n200 = Build Path(base path=w232, name or relative path=w236) -> (appended path=w235:path)
                        n201 = Write to Text File(file (use dialog)=w235, text=w239) -> (refnum out=w238:refnum<file>, error out=w237:errorcluster)  [unwired: 2 in, 1 out]
                        n202 = Close File(refnum=w238, error in=w237) -> ()  [unwired: 2 out]
                      }
                      frame True {
                      }
                    }
                    n203 = Build Array(TRUE, TRUE) -> (w227:bool[])
                    n204 = Build Array(FALSE) -> (w224:bool[])
                    n205 = local read "Fixed # of Frames"() -> (w222:u32)
                    n206 = call "DAQ Assistant"("data"=w227) -> ()  [unwired: 17 in, 2 out]
                    n207 = call "DAQ Assistant7"("data"=w224) -> ()  [unwired: 17 in, 2 out]
                    n208 = Initialize Array "Initialize Array"(nan, w222) -> (w220:dbl[])
                    n209 = while {
                      tunnel: w230 -> [w274]
                      tunnel: w229 -> [w273]
                      tunnel: w228 -> [_]
                      shift-right: [w245] -> _
                      shift-left: w220 -> [w246]
                      stop <- w247 stop-if-true
                      # "Only runs Real Time Fitting if \nReal Time Fitting box is checked \nand test function is off."
                      # "After testing is complete, turn off the lasers and\nreset  the buttons."
                      n210 = for {
                        N: 1 -> [_]
                        tunnel: w273 -> [w315]
                        tunnel: w274 -> [w314]
                        tunnel: [w311] -> w247
                        tunnel: [w310] -> w271
                        tunnel: [w308] -> w251
                        tunnel: [w307] -> w250
                        tunnel: [w306] -> w249
                        # "The logic here may look funny but it works elegantly. No matter if you choose \"Use Both Lasers\", the AND output is always\nfalse the first time these two boxes run since Laser 1 Value is always false, and the default is to use flow laser 1.\nBUT, the trick is if you chose \"Use Both Laser\" This big for loop is gonna run twice, the second time it runs, \nthe laser 1 value is TRUE because it is set to TRUE by the second box when the big for loop ran the first time. Now, when\nthe output of AND is true, ISS laser no longer runs. Only flow laser two is turned on and we execute the for loop to the right."
                        # "These two boxes take care of the flow chart.\nIt turn on ISS laser first, then triggers it and turn it off.\nIf ISS data is ready, then we go on to flow lase."
                        # "This loop may seem useless but it acts as a block. \nThis block does all the data collection, plotting and writing the data\nto file"
                        n211 = case shown="\"8 Detectors\", Default" w314 {
                          selector: w314 -> [w671 w672]
                          tunnel: [w671 w672] -> w312
                          frame "4 Detectors" {
                            n212 = dll-call lib="C:/Users/BUCKLEY-ADMIN/Desktop/DCScode_simulISS_MAP/flex05-4chPascal.dll" fn="USBStart" label="StartCH4"() -> ()  [unwired: 4 in, 2 out]
                          }
                          frame "8 Detectors", Default {
                            n213 = dll-call lib="C:/Users/BUCKLEY-ADMIN/Desktop/DCScode_simulISS_MAP/flex05oem8chauto100nsPASCAL_win7.dll" fn="USBStart" label="StartCH8"() -> ()  [unwired: 4 in, 2 out]
                          }
                        }
                        n214 = for {
                          N: 1 -> [_]
                          tunnel: w315 -> [w336]
                          tunnel: [w320] -> w311
                          tunnel: w312 -> [w325]
                          tunnel: [w328] -> w310
                          tunnel: "MARK\nMark" -> [w327]
                          tunnel: [w326] -> w308
                          tunnel: [w317] -> w307
                          tunnel: [w324] -> w306
                          w337 = FALSE
                          w346 = u8 2
                          # "Only saves data if\ntest function is off."
                          # "If Fixed # Frames check box is selected,\ncode will run for # of frames specified on \nfront panel and then call Stop button"
                          # "This for loop here acts as a block as well. It takes the relative \nflow data from UpdateData.vi and plot the data on the graph.\nWhen \"Baseline\" is selected,  the data point goes to 1. When\n\"Mark\" is selected, a point at positive infinity is plotted and a\nvertical line joining the point and the x axis if displayed."
                          n215 = while {
                            tunnel: [w527] -> w345
                            tunnel: [w497] -> w344
                            tunnel: [w498] -> w343
                            tunnel: [w501] -> w320
                            tunnel: [w528] -> w342
                            tunnel: w336 -> [w530]
                            tunnel: w325 -> [w503]
                            stop <- w532 stop-if-true
                            # "D4 Tail Alarm"
                            # "D2 Tail Alarm"
                            # "D8 Tail Alarm"
                            # "D7 Tail Alarm"
                            # "D6 Tail Alarm"
                            # "D5 Tail Alarm"
                            # "D3 Tail Alarm"
                            # "D1 Tail Alarm"
                            # "When press STOP, turn off DCS laser LED indicator is OFF"
                            n216 = Not(x="D4") -> (.not. x?=w516:bool)
                            n217 = Not(x="D8") -> (.not. x?=w512:bool)
                            n218 = Not(x="D5") -> (.not. x?=w515:bool)
                            n219 = Not(x="D1") -> (.not. x?=w519:bool)
                            n220 = Not(x="D6") -> (.not. x?=w514:bool)
                            n221 = Not(x="D2") -> (.not. x?=w504:bool)
                            n222 = Not(x="D7") -> (.not. x?=w513:bool)
                            n223 = Not(x="D3") -> (.not. x?=w517:bool)
                            n224 = case shown="True" "Stop" {
                              selector: "Stop" -> [w571 w577]
                              tunnel: [w571 w574] -> w501
                              frame False {
                              }
                              frame True {
                                n225 = call "Prompt User for Input"("Enable"=w577) -> ("Yes"=w574:bool)  [unwired: 17 in, 1 out]
                                n226 = Build Array(w574, FALSE) -> (w576:bool[])
                                n227 = call "DAQ Assistant2"("data"=w576) -> ()  [unwired: 17 in, 2 out]
                                n228 = local read "Laser Input Name"() -> (w572:refnum<visa-resource-name>)
                                n229 = call "iBs.vi"("Laser On/Off"=FALSE, "VISA resource name"=w572) -> ()
                              }
                            }
                            n230 = case shown="True" "Clear plots" {
                              frame False {
                              }
                              frame True {
                                n231 = invoke on="g2" class="XYGraph (strict)" method="Reinit To Default"() -> ()  [unwired: 3 in, 3 out]
                              }
                            }
                            n232 = case shown="False" w516 {
                              selector: w516 -> [w618 w623]
                              frame False {
                                n233 = property on="Tau 2" class="WFChart (strict)"("Active Plot"=u32 3) -> (error out=w620:errorcluster)  [unwired: 2 in, 1 out]
                                n234 = property on="g2" class="XYGraph (strict)"("Active Plot"=u32 3) -> (error out=w621:errorcluster)  [unwired: 2 in, 1 out]
                                n235 = property on="g2" class="XYGraph (strict)"(error in=w621, "Plot.Visible?"=w618) -> ()  [unwired: 1 in, 2 out]
                                n236 = property on="Tau 2" class="WFChart (strict)"(error in=w620, "Plot.Visible?"=w618) -> ()  [unwired: 1 in, 2 out]
                              }
                              frame True {
                                n237 = property on="Tau 2" class="WFChart (strict)"("Active Plot"=u32 3) -> (error out=w624:errorcluster)  [unwired: 2 in, 1 out]
                                n238 = property on="Tau 2" class="WFChart (strict)"(error in=w624, "Plot.Visible?"=w623) -> ()  [unwired: 1 in, 2 out]
                                n239 = property on="g2" class="XYGraph (strict)"("Active Plot"=u32 3) -> (error out=w626:errorcluster)  [unwired: 2 in, 1 out]
                                n240 = property on="g2" class="XYGraph (strict)"(error in=w626, "Plot.Visible?"=w623) -> ()  [unwired: 1 in, 2 out]
                              }
                            }
                            n241 = case shown="False" w512 {
                              selector: w512 -> [w578 w583]
                              frame False {
                                n242 = property on="Tau 2" class="WFChart (strict)"("Active Plot"=u32 7) -> (error out=w579:errorcluster)  [unwired: 2 in, 1 out]
                                n243 = property on="g2" class="XYGraph (strict)"("Active Plot"=u32 7) -> (error out=w581:errorcluster)  [unwired: 2 in, 1 out]
                                n244 = property on="g2" class="XYGraph (strict)"(error in=w581, "Plot.Visible?"=w578) -> ()  [unwired: 1 in, 2 out]
                                n245 = property on="Tau 2" class="WFChart (strict)"(error in=w579, "Plot.Visible?"=w578) -> ()  [unwired: 1 in, 2 out]
                              }
                              frame True {
                                n246 = property on="Tau 2" class="WFChart (strict)"("Active Plot"=u32 7) -> (error out=w585:errorcluster)  [unwired: 2 in, 1 out]
                                n247 = property on="Tau 2" class="WFChart (strict)"(error in=w585, "Plot.Visible?"=w583) -> ()  [unwired: 1 in, 2 out]
                                n248 = property on="g2" class="XYGraph (strict)"("Active Plot"=u32 7) -> (error out=w586:errorcluster)  [unwired: 2 in, 1 out]
                                n249 = property on="g2" class="XYGraph (strict)"(error in=w586, "Plot.Visible?"=w583) -> ()  [unwired: 1 in, 2 out]
                              }
                            }
                            n250 = case shown="False" w515 {
                              selector: w515 -> [w608 w613]
                              frame False {
                                n251 = property on="Tau 2" class="WFChart (strict)"("Active Plot"=u32 4) -> (error out=w610:errorcluster)  [unwired: 2 in, 1 out]
                                n252 = property on="g2" class="XYGraph (strict)"("Active Plot"=u32 4) -> (error out=w611:errorcluster)  [unwired: 2 in, 1 out]
                                n253 = property on="g2" class="XYGraph (strict)"(error in=w611, "Plot.Visible?"=w608) -> ()  [unwired: 1 in, 2 out]
                                n254 = property on="Tau 2" class="WFChart (strict)"(error in=w610, "Plot.Visible?"=w608) -> ()  [unwired: 1 in, 2 out]
                              }
                              frame True {
                                n255 = property on="Tau 2" class="WFChart (strict)"("Active Plot"=u32 4) -> (error out=w615:errorcluster)  [unwired: 2 in, 1 out]
                                n256 = property on="Tau 2" class="WFChart (strict)"(error in=w615, "Plot.Visible?"=w613) -> ()  [unwired: 1 in, 2 out]
                                n257 = property on="g2" class="XYGraph (strict)"("Active Plot"=u32 4) -> (error out=w616:errorcluster)  [unwired: 2 in, 1 out]
                                n258 = property on="g2" class="XYGraph (strict)"(error in=w616, "Plot.Visible?"=w613) -> ()  [unwired: 1 in, 2 out]
                              }
                            }
                            n259 = case shown="True" w519 {
                              selector: w519 -> [w648 w653]
                              frame False {
                                n260 = property on="Tau 2" class="WFChart (strict)"("Active Plot"=u32 0) -> (error out=w649:errorcluster)  [unwired: 2 in, 1 out]
                                n261 = property on="g2" class="XYGraph (strict)"("Active Plot"=u32 0) -> (error out=w651:errorcluster)  [unwired: 2 in, 1 out]
                                n262 = property on="g2" class="XYGraph (strict)"(error in=w651, "Plot.Visible?"=w648) -> ()  [unwired: 1 in, 2 out]
                                n263 = property on="Tau 2" class="WFChart (strict)"(error in=w649, "Plot.Visible?"=w648) -> ()  [unwired: 1 in, 2 out]
                              }
                              frame True {
                                n264 = property on="Tau 2" class="WFChart (strict)"("Active Plot"=u32 0) -> (error out=w655:errorcluster)  [unwired: 2 in, 1 out]
                                n265 = property on="Tau 2" class="WFChart (strict)"(error in=w655, "Plot.Visible?"=w653) -> ()  [unwired: 1 in, 2 out]
                                n266 = property on="g2" class="XYGraph (strict)"("Active Plot"=u32 0) -> (error out=w656:errorcluster)  [unwired: 2 in, 1 out]
                                n267 = property on="g2" class="XYGraph (strict)"(error in=w656, "Plot.Visible?"=w653) -> ()  [unwired: 1 in, 2 out]
                              }
                            }
                            n268 = case shown="False" w514 {
                              selector: w514 -> [w598 w603]
                              frame False {
                                n269 = property on="Tau 2" class="WFChart (strict)"("Active Plot"=u32 5) -> (error out=w600:errorcluster)  [unwired: 2 in, 1 out]
                                n270 = property on="g2" class="XYGraph (strict)"("Active Plot"=u32 5) -> (error out=w601:errorcluster)  [unwired: 2 in, 1 out]
                                n271 = property on="g2" class="XYGraph (strict)"(error in=w601, "Plot.Visible?"=w598) -> ()  [unwired: 1 in, 2 out]
                                n272 = property on="Tau 2" class="WFChart (strict)"(error in=w600, "Plot.Visible?"=w598) -> ()  [unwired: 1 in, 2 out]
                              }
                              frame True {
                                n273 = property on="Tau 2" class="WFChart (strict)"("Active Plot"=u32 5) -> (error out=w604:errorcluster)  [unwired: 2 in, 1 out]
                                n274 = property on="Tau 2" class="WFChart (strict)"(error in=w604, "Plot.Visible?"=w603) -> ()  [unwired: 1 in, 2 out]
                                n275 = property on="g2" class="XYGraph (strict)"("Active Plot"=u32 5) -> (error out=w606:errorcluster)  [unwired: 2 in, 1 out]
                                n276 = property on="g2" class="XYGraph (strict)"(error in=w606, "Plot.Visible?"=w603) -> ()  [unwired: 1 in, 2 out]
                              }
                            }
                            n277 = case shown="False" w504 {
                              selector: w504 -> [w638 w643]
                              frame False {
                                n278 = property on="Tau 2" class="WFChart (strict)"("Active Plot"=u32 1) -> (error out=w640:errorcluster)  [unwired: 2 in, 1 out]
                                n279 = property on="g2" class="XYGraph (strict)"("Active Plot"=u32 1) -> (error out=w641:errorcluster)  [unwired: 2 in, 1 out]
                                n280 = property on="g2" class="XYGraph (strict)"(error in=w641, "Plot.Visible?"=w638) -> ()  [unwired: 1 in, 2 out]
                                n281 = property on="Tau 2" class="WFChart (strict)"(error in=w640, "Plot.Visible?"=w638) -> ()  [unwired: 1 in, 2 out]
                              }
                              frame True {
                                n282 = property on="Tau 2" class="WFChart (strict)"("Active Plot"=u32 1) -> (error out=w645:errorcluster)  [unwired: 2 in, 1 out]
                                n283 = property on="Tau 2" class="WFChart (strict)"(error in=w645, "Plot.Visible?"=w643) -> ()  [unwired: 1 in, 2 out]
                                n284 = property on="g2" class="XYGraph (strict)"("Active Plot"=u32 1) -> (error out=w646:errorcluster)  [unwired: 2 in, 1 out]
                                n285 = property on="g2" class="XYGraph (strict)"(error in=w646, "Plot.Visible?"=w643) -> ()  [unwired: 1 in, 2 out]
                              }
                            }
                            n286 = case shown="False" w513 {
                              selector: w513 -> [w588 w593]
                              frame False {
                                n287 = property on="Tau 2" class="WFChart (strict)"("Active Plot"=u32 6) -> (error out=w590:errorcluster)  [unwired: 2 in, 1 out]
                                n288 = property on="g2" class="XYGraph (strict)"("Active Plot"=u32 6) -> (error out=w591:errorcluster)  [unwired: 2 in, 1 out]
                                n289 = property on="g2" class="XYGraph (strict)"(error in=w591, "Plot.Visible?"=w588) -> ()  [unwired: 1 in, 2 out]
                                n290 = property on="Tau 2" class="WFChart (strict)"(error in=w590, "Plot.Visible?"=w588) -> ()  [unwired: 1 in, 2 out]
                              }
                              frame True {
                                n291 = property on="Tau 2" class="WFChart (strict)"("Active Plot"=u32 6) -> (error out=w594:errorcluster)  [unwired: 2 in, 1 out]
                                n292 = property on="Tau 2" class="WFChart (strict)"(error in=w594, "Plot.Visible?"=w593) -> ()  [unwired: 1 in, 2 out]
                                n293 = property on="g2" class="XYGraph (strict)"("Active Plot"=u32 6) -> (error out=w596:errorcluster)  [unwired: 2 in, 1 out]
                                n294 = property on="g2" class="XYGraph (strict)"(error in=w596, "Plot.Visible?"=w593) -> ()  [unwired: 1 in, 2 out]
                              }
                            }
                            n295 = case shown="False" w517 {
                              selector: w517 -> [w628 w633]
                              frame False {
                                n296 = property on="Tau 2" class="WFChart (strict)"("Active Plot"=u32 2) -> (error out=w629:errorcluster)  [unwired: 2 in, 1 out]
                                n297 = property on="g2" class="XYGraph (strict)"("Active Plot"=u32 2) -> (error out=w631:errorcluster)  [unwired: 2 in, 1 out]
                                n298 = property on="g2" class="XYGraph (strict)"(error in=w631, "Plot.Visible?"=w628) -> ()  [unwired: 1 in, 2 out]
                                n299 = property on="Tau 2" class="WFChart (strict)"(error in=w629, "Plot.Visible?"=w628) -> ()  [unwired: 1 in, 2 out]
                              }
                              frame True {
                                n300 = property on="Tau 2" class="WFChart (strict)"("Active Plot"=u32 2) -> (error out=w635:errorcluster)  [unwired: 2 in, 1 out]
                                n301 = property on="Tau 2" class="WFChart (strict)"(error in=w635, "Plot.Visible?"=w633) -> ()  [unwired: 1 in, 2 out]
                                n302 = property on="g2" class="XYGraph (strict)"("Active Plot"=u32 2) -> (error out=w636:errorcluster)  [unwired: 2 in, 1 out]
                                n303 = property on="g2" class="XYGraph (strict)"(error in=w636, "Plot.Visible?"=w633) -> ()  [unwired: 1 in, 2 out]
                              }
                            }
                            n304 = Wait (ms)(milliseconds to wait="Update Time (ms)\nDO NOT CHANGE!") -> ()  [unwired: 1 out]
                            n305 = call "UpdateData.vi"("Duration Time (ms)"="Integration Time (ms)", "Detector Select"=w503, "Delay Time"=w530) -> ("Elapsed Time(s)"=w531:sgl, "Intensity Array"=w529:sgl[], "Tau Array"=w528:sgl[], "mean"=w493:dbl, "mean 8"=w473:dbl, "mean 2"=w442:dbl, "mean 7"=w474:dbl, "mean 3"=w478:dbl, "Intensity data"=w527:string, "g2 Display"=→"g2":cluster{"Delay Time":sgl[], sgl[]}[], "mean 4"=w477:dbl, "mean 5"=w476:dbl, "mean 6"=w475:dbl, "tau data"=w497:string, "g2 data"=w498:string)  [unwired: 2 in]
                            n306 = Multiply(x=sgl 1000.0, y=w531) -> (x*y=w535:sgl)
                            n307 = Less?(x=w493, y=1.005) -> (x < y?=w472:bool)
                            n308 = Less?(x=w442, y=1.005) -> (x < y?=w426:bool)
                            n309 = Less?(x=w478, y=1.005) -> (x < y?=w425:bool)
                            n310 = Less?(x=w477, y=1.005) -> (x < y?=w422:bool)
                            n311 = Less?(x=w476, y=1.005) -> (x < y?=w420:bool)
                            n312 = Less?(x=w475, y=1.005) -> (x < y?=w418:bool)
                            n313 = Less?(x=w474, y=1.005) -> (x < y?=w416:bool)
                            n314 = Less?(x=w473, y=1.005) -> (x < y?=w414:bool)
                            n315 = Index Array(array=w529, index #1=0, index #2=1, index #3=2, index #4=3, index #5=4, index #6=5, index #7=6, index #8=7) -> (element #1=w470:sgl, element #2=w449:sgl, element #3=w448:sgl, element #4=w447:sgl, element #5=w446:sgl, element #6=w445:sgl, element #7=w444:sgl, element #8=w443:sgl)
                            "Det 7" <- w444
                            "Det 6" <- w445
                            "Det 5" <- w446
                            "Det 4" <- w447
                            "Det 3" <- w448
                            "Det 2" <- w449
                            "Det 1" <- w470
                            "Det 8" <- w443
                            n316 = Subtract(x="Integration Time (ms)", y=w535) -> (x-y=w533:sgl)
                            "Time Left (ms)" <- w533
                            n317 = Greater?(x=w493, y=0.98) -> (0:w471:bool)
                            n318 = Greater?(x=w477, y=0.98) -> (0:w423:bool)
                            n319 = Greater?(x=w475, y=0.98) -> (0:w419:bool)
                            n320 = Greater?(x=w473, y=0.98) -> (0:w415:bool)
                            n321 = Greater Or Equal?(x=w470, y=sgl 2.0) -> (x >= y?=w467:bool)
                            n322 = Greater Or Equal?(x=w449, y=sgl 2.0) -> (x >= y?=w413:bool)
                            n323 = Greater Or Equal?(x=w448, y=sgl 2.0) -> (x >= y?=w411:bool)
                            n324 = Greater Or Equal?(x=w447, y=sgl 2.0) -> (x >= y?=w409:bool)
                            n325 = Greater Or Equal?(x=w446, y=sgl 2.0) -> (x >= y?=w407:bool)
                            n326 = Greater Or Equal?(x=w445, y=sgl 2.0) -> (x >= y?=w405:bool)
                            n327 = Less Or Equal?(x=w470, y=sgl 1000.0) -> (x <= y?=w466:bool)
                            n328 = Less Or Equal?(x=w449, y=sgl 1000.0) -> (x <= y?=w412:bool)
                            n329 = Less Or Equal?(x=w448, y=sgl 1000.0) -> (x <= y?=w410:bool)
                            n330 = Less Or Equal?(x=w447, y=sgl 1000.0) -> (x <= y?=w408:bool)
                            n331 = Less Or Equal?(x=w446, y=sgl 1000.0) -> (x <= y?=w406:bool)
                            n332 = Less Or Equal?(x=w445, y=sgl 1000.0) -> (x <= y?=w404:bool)
                            n333 = Less Or Equal?(x=w444, y=sgl 1000.0) -> (x <= y?=w402:bool)
                            n334 = Less Or Equal?(x=w443, y=sgl 1000.0) -> (x <= y?=w400:bool)
                            n335 = Greater Or Equal?(x=w444, y=sgl 2.0) -> (x >= y?=w403:bool)
                            n336 = Greater Or Equal?(x=w443, y=sgl 2.0) -> (x >= y?=w401:bool)
                            n337 = Greater?(x=w442, y=0.98) -> (0:w427:bool)
                            n338 = Greater?(x=w478, y=0.98) -> (0:w424:bool)
                            n339 = Greater?(x=w476, y=0.98) -> (0:w421:bool)
                            n340 = Greater?(x=w474, y=0.98) -> (0:w417:bool)
                            n341 = Build Array(w472, w471, w467, w466) -> (w465:bool[])
                            n342 = Build Array(w427, w426, w413, w412) -> (w441:bool[])
                            n343 = Build Array(w425, w424, w411, w410) -> (w440:bool[])
                            n344 = Build Array(w423, w422, w409, w408) -> (w439:bool[])
                            n345 = Build Array(w421, w420, w407, w406) -> (w438:bool[])
                            n346 = Build Array(w419, w418, w405, w404) -> (w437:bool[])
                            n347 = Build Array(w417, w416, w403, w402) -> (w436:bool[])
                            n348 = Build Array(w415, w414, w401, w400) -> (w435:bool[])
                            n349 = And Array Elements(Boolean array=w465) -> (logical AND=w464:bool)
                            n350 = And Array Elements(Boolean array=w441) -> (logical AND=w428:bool)
                            n351 = And Array Elements(Boolean array=w440) -> (logical AND=w429:bool)
                            n352 = And Array Elements(Boolean array=w439) -> (logical AND=w430:bool)
                            n353 = And Array Elements(Boolean array=w438) -> (logical AND=w431:bool)
                            n354 = And Array Elements(Boolean array=w437) -> (logical AND=w432:bool)
                            n355 = And Array Elements(Boolean array=w436) -> (logical AND=w433:bool)
                            n356 = And Array Elements(Boolean array=w435) -> (logical AND=w434:bool)
                            n357 = Less Or Equal To 0?(x=w533) -> (x <= 0?=w534:bool)
                            n358 = case shown="True" w464 {
                              frame False {
                                n359 = control-ref of="Det 1"() -> (w567:refnum<vi>)
                                n360 = property on="Property Node" class="Digital (strict)"(reference=w567, "DisabledEnum"=T5."Disabled and Grayed Out" ("Disabled")) -> ()  [unwired: 1 in, 2 out]
                              }
                              frame True {
                                n361 = control-ref of="Det 1"() -> (w569:refnum<vi>)
                                n362 = property on="Property Node" class="Digital (strict)"(reference=w569, "DisabledEnum"=T5."Enabled" ("Disabled")) -> ()  [unwired: 1 in, 2 out]
                              }
                            }
                            n363 = case shown="True" w428 {
                              frame False {
                                n364 = control-ref of="Det 2"() -> (w563:refnum<vi>)
                                n365 = property on="Property Node" class="Digital (strict)"(reference=w563, "DisabledEnum"=T5."Disabled and Grayed Out" ("Disabled")) -> ()  [unwired: 1 in, 2 out]
                              }
                              frame True {
                                n366 = control-ref of="Det 2"() -> (w565:refnum<vi>)
                                n367 = property on="Property Node" class="Digital (strict)"(reference=w565, "DisabledEnum"=T5."Enabled" ("Disabled")) -> ()  [unwired: 1 in, 2 out]
                              }
                            }
                            n368 = case shown="True" w429 {
                              frame False {
                                n369 = control-ref of="Det 3"() -> (w559:refnum<vi>)
                                n370 = property on="Property Node" class="Digital (strict)"(reference=w559, "DisabledEnum"=T5."Disabled and Grayed Out" ("Disabled")) -> ()  [unwired: 1 in, 2 out]
                              }
                              frame True {
                                n371 = control-ref of="Det 3"() -> (w561:refnum<vi>)
                                n372 = property on="Property Node" class="Digital (strict)"(reference=w561, "DisabledEnum"=T5."Enabled" ("Disabled")) -> ()  [unwired: 1 in, 2 out]
                              }
                            }
                            n373 = case shown="True" w430 {
                              frame False {
                                n374 = control-ref of="Det 4"() -> (w555:refnum<vi>)
                                n375 = property on="Property Node" class="Digital (strict)"(reference=w555, "DisabledEnum"=T5."Disabled and Grayed Out" ("Disabled")) -> ()  [unwired: 1 in, 2 out]
                              }
                              frame True {
                                n376 = control-ref of="Det 4"() -> (w557:refnum<vi>)
                                n377 = property on="Property Node" class="Digital (strict)"(reference=w557, "DisabledEnum"=T5."Enabled" ("Disabled")) -> ()  [unwired: 1 in, 2 out]
                              }
                            }
                            n378 = case shown="True" w431 {
                              frame False {
                                n379 = control-ref of="Det 5"() -> (w551:refnum<vi>)
                                n380 = property on="Property Node" class="Digital (strict)"(reference=w551, "DisabledEnum"=T5."Disabled and Grayed Out" ("Disabled")) -> ()  [unwired: 1 in, 2 out]
                              }
                              frame True {
                                n381 = control-ref of="Det 5"() -> (w553:refnum<vi>)
                                n382 = property on="Property Node" class="Digital (strict)"(reference=w553, "DisabledEnum"=T5."Enabled" ("Disabled")) -> ()  [unwired: 1 in, 2 out]
                              }
                            }
                            n383 = case shown="False" w432 {
                              frame False {
                                n384 = control-ref of="Det 6"() -> (w547:refnum<vi>)
                                n385 = property on="Property Node" class="Digital (strict)"(reference=w547, "DisabledEnum"=T5."Disabled and Grayed Out" ("Disabled")) -> ()  [unwired: 1 in, 2 out]
                              }
                              frame True {
                                n386 = control-ref of="Det 6"() -> (w549:refnum<vi>)
                                n387 = property on="Property Node" class="Digital (strict)"(reference=w549, "DisabledEnum"=T5."Enabled" ("Disabled")) -> ()  [unwired: 1 in, 2 out]
                              }
                            }
                            n388 = case shown="True" w433 {
                              frame False {
                                n389 = control-ref of="Det 7"() -> (w543:refnum<vi>)
                                n390 = property on="Property Node" class="Digital (strict)"(reference=w543, "DisabledEnum"=T5."Disabled and Grayed Out" ("Disabled")) -> ()  [unwired: 1 in, 2 out]
                              }
                              frame True {
                                n391 = control-ref of="Det 7"() -> (w545:refnum<vi>)
                                n392 = property on="Property Node" class="Digital (strict)"(reference=w545, "DisabledEnum"=T5."Enabled" ("Disabled")) -> ()  [unwired: 1 in, 2 out]
                              }
                            }
                            n393 = case shown="True" w434 {
                              frame False {
                                n394 = control-ref of="Det 8"() -> (w539:refnum<vi>)
                                n395 = property on="Property Node" class="Digital (strict)"(reference=w539, "DisabledEnum"=T5."Disabled and Grayed Out" ("Disabled")) -> ()  [unwired: 1 in, 2 out]
                              }
                              frame True {
                                n396 = control-ref of="Det 8"() -> (w541:refnum<vi>)
                                n397 = property on="Property Node" class="Digital (strict)"(reference=w541, "DisabledEnum"=T5."Enabled" ("Disabled")) -> ()  [unwired: 1 in, 2 out]
                              }
                            }
                            n398 = Or(x=w501, y=w534) -> (x .or. y?=w532:bool)
                            n399 = case shown="True" w532 {
                              tunnel: w503 -> [w658 _]
                              frame True {
                                n400 = case shown="\"8 Detectors\", Default" w658 {
                                frame "4 Detectors" {
                                n401 = dll-call lib="C:/Users/BUCKLEY-ADMIN/Desktop/DCScode_simulISS_MAP/flex05-4chPascal.dll" fn="USBStop" label="StopCH4"() -> ()  [unwired: 4 in, 2 out]
                                }
                                frame "8 Detectors", Default {
                                n402 = dll-call lib="C:/Users/BUCKLEY-ADMIN/Desktop/DCScode_simulISS_MAP/flex05oem8chauto100nsPASCAL_win7.dll" fn="USBStop" label="StopCH8"() -> ()  [unwired: 4 in, 2 out]
                                }
                                }
                              }
                              frame False {
                              }
                            }
                          }
                          n403 = Current VI's Menubar() -> (w339:refnum<k9>)
                          n404 = local read "Trial #"() -> (w332:u32)
                          n405 = property on="QUIT" class="Bool (strict)"("Disabled"=w346) -> ()  [unwired: 2 in, 2 out]
                          n406 = Set Menu Item Info(7:"File", 9:w337, 11:w339) -> (3:w338:refnum<k9>)  [unwired: 4 in, 1 out]
                          n407 = Increment(x=w332) -> (x+1=w331:u32)
                          n408 = property on="Sequence Scan" class="Bool"("Disabled"=w346) -> ()  [unwired: 2 in, 2 out]
                          n409 = property on="Update Time (ms)\nDO NOT CHANGE!" class="DigNum (strict)"("Disabled"=w346) -> ()  [unwired: 2 in, 2 out]
                          n410 = property on="Integration Time (ms)" class="DigNum (strict)"("Disabled"=w346) -> ()  [unwired: 2 in, 2 out]
                          n411 = property on="Detector Select" class="RadioBtnsControl (strict)"("Disabled"=w346) -> ()  [unwired: 2 in, 2 out]
                          n412 = property on="Initialize Correlator" class="Bool"("Disabled"=w346) -> ()  [unwired: 2 in, 2 out]
                          n413 = local write "Trial #"(w331) -> ()
                          n414 = Set Menu Item Info(7:"Options", 9:w337, 11:w338) -> ()  [unwired: 4 in, 2 out]
                          n415 = case shown="\"Det 2\"" "Detector Used" {
                            tunnel: [1 2 3 4 5 6 7 8] -> w334
                            frame "Det 1", Default {
                            }
                            frame "Det 2" {
                            }
                            frame "Det 3" {
                            }
                            frame "Det 4" {
                            }
                            frame "Det 5" {
                            }
                            frame "Det 6" {
                            }
                            frame "Det 7" {
                            }
                            frame "Det 8" {
                            }
                          }
                          n416 = for {
                            N: 1 -> [_]
                            tunnel: w342 -> [w388]
                            tunnel: [w391] -> w335
                            tunnel: w334 -> [w390]
                            tunnel: w327 -> [w381]
                            n417 = case shown="True" w381 {
                              tunnel: [u32 0 w397] -> w391
                              frame False {
                              }
                              frame True {
                                n418 = local write "Trial #"(u32 0) -> ()
                                n419 = local read "Mark #"() -> (w399:u32)
                                n420 = Increment(x=w399) -> (x+1=w397:u32)
                                n421 = local write "Mark #"(w397) -> ()
                              }
                            }
                            n422 = Index Array(array=w388, index=w390) -> (element=w389:sgl)
                            n423 = Boolean To (0,1)(Boolean="Baseline") -> (0, 1=w393:i16)
                            n424 = case shown="False" w381 {
                              tunnel: [0.0 w395] -> w385
                              tunnel: inf -> [_ w395]
                              frame False {
                              }
                              frame True {
                              }
                            }
                            n425 = feedback #1() -> (w386:sgl)  [unwired: 1 in]
                            n426 = formula code="if(Tau==0) Tau=Tau+0.001;\nif(T==1) baselineflow=Tau;\n\ntmp=baselineflow/Tau;"("Tau"=w389, "T"=w393, "baselineflow"=w386) -> ("tmp"=w383:dbl, "baselineflow"=w387:sgl)
                            n427 = feedback-in #1(w387) -> ()
                            n428 = Bundle("tmp"=w383, w385) -> (→"Tau":cluster{"tmp":dbl, dbl})  [unwired: 1 in]
                          }
                          n429 = property on="Frame #" class="DigNum (strict)"() -> ("Value"=w318:u32)  [unwired: 2 in, 2 out]
                          n430 = case shown="True" "Fixed Time" {
                            tunnel: w318 -> [w369 w372]
                            tunnel: [w369 w372] -> w317
                            frame False {
                            }
                            frame True {
                              n431 = Less Or Equal?(x="Fixed # of Frames", y=w372) -> (x <= y?=w370:bool)
                              n432 = local write "Stop"(w370) -> ()
                            }
                          }
                          n433 = case shown="\"8 Detectors\", Default" w325 {
                            tunnel: w335 -> [w666 w670]
                            tunnel: [w667 w669] -> w352
                            tunnel: [4 8] -> w324
                            frame "4 Detectors" {
                              n434 = Build Array(w666, w666, w666, w666, w666) -> (w667:u32[])
                            }
                            frame "8 Detectors", Default {
                              n435 = Build Array(w670, w670, w670, w670, w670, w670, w670, w670, w670) -> (w669:u32[])
                            }
                          }
                          n436 = case shown="\"8 Detectors\", Default" w325 {
                            tunnel: ["%Duration\tID1\t\tID2\t\tID3\t\tID4\n" "%Duration\tID1\t\tID2\t\tID3\t\tID4\t\tID5\t\tID6\t\tID7\t\tID8\n"] -> w349
                            tunnel: ["%Tau\t\tTau1\t\tTau2\t\tTau3\t\tTau4\n" "%Tau\t\tTau1\t\tTau2\t\tTau3\t\tTau4\t\tTau5\t\tTau6\t\tTau7\t\tTau8\n"] -> w348
                            tunnel: ["%Delaytime\tD1\t\tD2\t\tD3\t\tD4\n" "%Delaytime\tD1\t\tD2\t\tD3\t\tD4\t\tD5\t\tD6\t\tD7\t\tD8\n"] -> w347
                            frame "4 Detectors" {
                            }
                            frame "8 Detectors", Default {
                            }
                          }
                          n437 = Increment(x=w317) -> (x+1=w319:u32)
                          n438 = Number To Decimal String(number=w317) -> (decimal integer string=w353:string)  [unwired: 1 in]
                          n439 = local write "Frame #"(w319) -> ()
                          n440 = Get Date/Time In Seconds() -> (seconds since 1Jan1904=w362:timestamp)
                          n441 = Array To Spreadsheet String(array=w352, 3:"%d") -> (spreadsheet string=w350:string)  [unwired: 1 in]
                          n442 = Format Date/Time String(seconds (now)=w362) -> (date/time string=w359:string)  [unwired: 2 in]
                          "Computer Time" <- w359
                          n443 = Concatenate Strings("File\nName:", "_flow_", w353, ".dat") -> (w322:string)
                          n444 = local read "Test"() -> (w316:bool)
                          n445 = Concatenate Strings("%", w359, "\r\n", w349, w345, w348, "%\t\t", w344, w347, w343, w350) -> (w330:string)
                          n446 = Build Path(base path="Data Save Directory:", name or relative path=w322) -> (appended path=w329:path)
                          n447 = case shown="False" w316 {
                            tunnel: w330 -> [w366 _]
                            tunnel: w329 -> [w365 _]
                            tunnel: [w364 _] -> w328
                            tunnel: [w363 _] -> w326
                            frame False {
                              n448 = Write to Text File(file (use dialog)=w365, text=w366) -> (refnum out=w367:refnum<file>, error out=w368:errorcluster)  [unwired: 2 in, 1 out]
                              n449 = Close File(refnum=w367, error in=w368) -> (path=w364:path, error out=w363:errorcluster)
                            }
                            frame True {
                            }
                          }
                        }
                      }
                      n450 = Index Array(array="Visible Averages", index=3) -> (element=w265:bool)
                      n451 = Index Array(array="Visible Averages", index=1) -> (element=w266:bool)
                      n452 = Index Array(array="Visible Averages", index=0) -> (element=w259:bool)
                      n453 = Index Array(array="Visible Averages", index=2) -> (element=w260:bool)
                      n454 = property on="Tau 2" class="WFChart (strict)"("Active Plot"=u32 11) -> (error out=w263:errorcluster)  [unwired: 2 in, 1 out]
                      n455 = property on="Tau 2" class="WFChart (strict)"("Active Plot"=u32 9) -> (error out=w268:errorcluster)  [unwired: 2 in, 1 out]
                      n456 = property on="Tau 2" class="WFChart (strict)"("Active Plot"=u32 8) -> (error out=w257:errorcluster)  [unwired: 2 in, 1 out]
                      n457 = property on="Tau 2" class="WFChart (strict)"("Active Plot"=u32 10) -> (error out=w262:errorcluster)  [unwired: 2 in, 1 out]
                      n458 = property on="Tau 2" class="WFChart (strict)"(error in=w263, "Plot.Visible?"=w265) -> ()  [unwired: 1 in, 2 out]
                      n459 = property on="Tau 2" class="WFChart (strict)"(error in=w268, "Plot.Visible?"=w266) -> ()  [unwired: 1 in, 2 out]
                      n460 = property on="Tau 2" class="WFChart (strict)"(error in=w257, "Plot.Visible?"=w259) -> ()  [unwired: 1 in, 2 out]
                      n461 = property on="Tau 2" class="WFChart (strict)"(error in=w262, "Plot.Visible?"=w260) -> ()  [unwired: 1 in, 2 out]
                      n462 = local read "Test"() -> (w243:bool)
                      n463 = Not(x=w243) -> (.not. x?=w242:bool)
                      n464 = Unbundle By Name(w251) -> ("status"=w270:bool)
                      n465 = for {
                        N: 1 -> [_]
                        tunnel: w271 -> [_]
                        n466 = local write "Stop"(FALSE) -> ()
                        n467 = Wait (ms)(milliseconds to wait="Delay between frames(ms)") -> ()  [unwired: 1 out]
                      }
                      n468 = And(x="Real Time Fitting?", y=w242) -> (x .and. y?=w241:bool)
                      n469 = Not(x=w270) -> (.not. x?=w269:bool)
                      n470 = case shown="True" w241 {
                        tunnel: w269 -> [_ w280]
                        tunnel: w250 -> [_ w279]
                        tunnel: w249 -> [_ w278]
                        tunnel: w246 -> [w275 w277]
                        tunnel: [w275 w276] -> w245
                        frame False {
                        }
                        frame True {
                          n471 = case shown="True" w280 {
                            tunnel: w279 -> [_ w300]
                            tunnel: w278 -> [_ w296]
                            tunnel: w277 -> [w281 w292]
                            tunnel: [w281 w290] -> w276
                            frame False {
                            }
                            frame True {
                              # "Initialize Array of NaNs with size of \"fixed number of frames, \nand run this array into the case structure by putting it \nthrough a shift register with each loop it will replace one of \nthe NaNs by the flow data of the detector used. Then this data\nis averaged and COV is calculated."
                              n472 = property on="Data Save Directory:" class="Path"() -> ("Value"=w302:path)  [unwired: 2 in, 2 out]
                              n473 = property on="File\nName:" class="Str"() -> ("Value"=w303:string)  [unwired: 2 in, 2 out]
                              n474 = call "GetFilePath.vi"("path"=w302, "file name"=w303, "frame number"=w300) -> ("final path C"=w295:string)  [unwired: 10 in, 2 out]
                              n475 = property on="Avg" class="Arr (strict)"() -> ("Value"=w301:bool[][])  [unwired: 2 in, 2 out]
                              n476 = call "DCSAnalysis.vi"("# Detectors"=w296, "File path"=w295, "Frame #"=w300, "rho"="rho", "other settings"="Other Settings", "avgBool"=w301, "var values"="Initial Guess") -> ("Flow in each detector"=w293:dbl[], "Tau"=→"Tau 2":T3)  [unwired: 18 in, 1 out]
                              "Flow in each detector" <- w293
                              n477 = local read "Detector Used"() -> (w282:T2)
                              n478 = local read "Trial #"() -> (w288:u32)
                              n479 = Decrement(x=w288) -> (x-1=w289:u32)
                              n480 = Index Array(array=w293, index=w282) -> (element=w291:dbl)
                              n481 = Replace Array Subset(array=w292, new element=w291, index=w289) -> (w290:dbl[])
                              n482 = call <vilib>:"Std Deviation and Variance.vi"("X"=w290) -> ("mean"=w286:dbl, "standard deviation"=w287:dbl)  [unwired: 1 in, 1 out]
                              "mean" <- w286
                              n483 = Divide(x=w287, y=w286) -> (x/y=w284:dbl)
                              n484 = Multiply(x=w284, y=100.0) -> (x*y=→"COV":dbl)
                            }
                          }
                        }
                      }
                    }
                    n485 = call "iBs.vi"("Laser On/Off"=TRUE, "VISA resource name"="Laser Input Name") -> ()
                  }
                  frame True {
                    n486 = invoke on="Sequence Scan" class="Bool" method="Reinit To Default"() -> ()  [unwired: 3 in, 3 out]
                    n487 = call "Display Message to User5"() -> ()  [unwired: 10 in, 2 out]
                  }
                }
              }
            }
            "Frame #" <- u32 0
            "Mark #" <- u32 0
            "Trial #" <- u32 0
          }
          event "QUIT": Value Change {
            # "Reset correlator before quitting"
            n488 = event-data() -> ()  [unwired: 1 in, 6 out]
            n489 = case shown="\"8 Detectors\", Default" w678 {
              frame "4 Detectors" {
                n490 = dll-call lib="C:/Users/BUCKLEY-ADMIN/Desktop/DCScode_simulISS_MAP/flex05-4chPascal.dll" fn="USBInitialize" label="InitCH4"() -> (error out=w680:errorcluster)  [unwired: 4 in, 1 out]
                n491 = dll-call lib="C:/Users/BUCKLEY-ADMIN/Desktop/DCScode_simulISS_MAP/flex05-4chPascal.dll" fn="USBFree" label="FreeCH4"(error in=w680) -> ()  [unwired: 3 in, 2 out]
              }
              frame "8 Detectors", Default {
                n492 = dll-call lib="C:/Users/BUCKLEY-ADMIN/Desktop/DCScode_simulISS_MAP/flex05oem8chauto100nsPASCAL_win7.dll" fn="USBInitialize" label="InitCH8"() -> (error out=w681:errorcluster)  [unwired: 4 in, 1 out]
                n493 = dll-call lib="C:/Users/BUCKLEY-ADMIN/Desktop/DCScode_simulISS_MAP/flex05oem8chauto100nsPASCAL_win7.dll" fn="USBFree" label="FreeCH8"(error in=w681) -> ()  [unwired: 3 in, 2 out]
              }
            }
            n494 = local write "Status"("Quit") -> ()
            n495 = local write "Status"("Quit") -> ()
          }
          event Timeout {
            w686 = TRUE
            w685 = u8 0
            # "This case structure turns on\n      and off the ISS Lasers"
            # "This case structure ensures that when the\noptical switch is turned on, the relay tells \nthe laser to power on."
            # "The system sits here and wait for some buttons to be pressed. And the status is always \"waiting\". Once some button is pressed, this value driven event\nstructure goes to the appropriate frame."
            n496 = event-data() -> ()  [unwired: 1 in, 3 out]
            n497 = local write "Status"("Waiting") -> ()
            n498 = property on="MARK\nMark" class="Bool"("DisabledEnum"=w685) -> ()  [unwired: 2 in, 2 out]
            n499 = property on="QUIT" class="Bool (strict)"("Disabled"=w685) -> ()  [unwired: 2 in, 2 out]
            n500 = property on="Sequence Scan" class="Bool"("Disabled"=w685) -> ()  [unwired: 2 in, 2 out]
            n501 = property on="Initialize Correlator" class="Bool"("Disabled"=w685) -> ()  [unwired: 2 in, 2 out]
            n502 = property on="Update Time (ms)\nDO NOT CHANGE!" class="DigNum (strict)"("Disabled"=w685) -> ()  [unwired: 2 in, 2 out]
            n503 = property on="Integration Time (ms)" class="DigNum (strict)"("Disabled"=w685) -> ()  [unwired: 2 in, 2 out]
            n504 = property on="Detector Select" class="RadioBtnsControl (strict)"("Disabled"=w685) -> ()  [unwired: 2 in, 2 out]
            n505 = case shown="True" "ISS Lasers ON" {
              frame False {
                n506 = Build Array(FALSE) -> (w693:bool[])
                n507 = call "DAQ Assistant5"("data"=w693) -> ()  [unwired: 17 in, 2 out]
              }
              frame True {
                # "For Toptica laser control"
                n508 = local read "Laser Input Name"() -> (w695:refnum<visa-resource-name>)
                n509 = call "iBs.vi"("Laser On/Off"=TRUE, "VISA resource name"=w695) -> ()
                n510 = Build Array(TRUE) -> (w697:bool[])
                n511 = call "DAQ Assistant6"("data"=w697) -> ()  [unwired: 17 in, 2 out]
              }
            }
            n512 = case shown="True" "Optical Switch OPEN" {
              frame False {
                # "Send 2 signals, one for LED indicator, one for switch"
                n513 = Build Array(FALSE, FALSE) -> (w699:bool[])
                n514 = call "DAQ Assistant3"("data"=w699) -> ()  [unwired: 17 in, 2 out]
              }
              frame True {
                n515 = Build Array(TRUE, TRUE) -> (w702:bool[])
                n516 = call "DAQ Assistant4"("data"=w702) -> ()  [unwired: 17 in, 2 out]
              }
            }
            n517 = Current VI's Menubar() -> (w688:refnum<k9>)
            n518 = Set Menu Item Info(7:"File", 9:w686, 11:w688) -> (3:w687:refnum<k9>)  [unwired: 4 in, 1 out]
            n519 = Get Date/Time In Seconds() -> (seconds since 1Jan1904=w691:timestamp)
            n520 = Set Menu Item Info(7:"Options", 9:w686, 11:w687) -> ()  [unwired: 4 in, 2 out]
            n521 = Format Date/Time String(seconds (now)=w691) -> (date/time string=w692:string)  [unwired: 2 in]
            n522 = local write "Computer Time"(w692) -> ()
          }
        }
      }
    }
  }
  "Trial In Progress" <- FALSE ("Trial In Progress")
